vi "UHR-Fleezers Control (fpga) - 11.7.1UCBMeng5RG3.vi"() -> ()   [LabVIEW 2014]
doc: "UHR-Fleezers Instrument Control Code (fpga)"
uses:
  <vilib>/Platform/TimedLoop/XDataNode/timing_clust.ctl
  <vilib>/Platform/TimedLoop/XDataNode/nitl_modes.ctl
  <vilib>/Platform/TimedLoop/XDataNode/wakeup.ctl
  <vilib>/rvi/Emulation/niFpgaGetClockAttributes.vi
  <vilib>/rvi/Emulation/niFpgaSctlEmulationGetInTimedLoop.vi
  <vilib>/rvi/Emulation/niFpgaEmulationReportErrorSimple.vi
  <vilib>/rvi/Emulation/niFpgaProcessEmulError.vi
  <vilib>/rvi/eio/common/nirviEmuTemplateMethod_errors.vi
  <vilib>/rvi/Emulation/niFpgaCriticalErrorInLSC.vi
  <vilib>/rvi/interface/RandomDataEmulation/niFpgaRandomDataHandleErrors.vi
  <vilib>/eio/EIONode/EIONode.xnode
  <vilib>/eio/EIOMethodNode/EIOMethodNode.xnode
  <vilib>/rvi/DataTransferAndStorage/Container/XNode/niFpgaContainer.xnode
  <vilib>/rvi/interface/RandomDataEmulation/nirviRandomDataFpgaReadWriteTemplate.vi
  <vilib>/addons/control/pid/fpga.llb/XNode/niFpgaPID.xnode
  <vilib>/Platform/TimedLoop/XDataNode/XDataNode.xnode
  <vilib>/Platform/TimedLoop/XDataNode/XDNodeRunTimeDep.lvlib
panel:
  in  "Tab Control":T1(tab)=enum."Force FB"
  in  "Set 3":bool
  in  "Set 2":bool=TRUE
  in  "Set 1":bool=TRUE
  in  "Trap Pos to FIFO":bool
  in  "N of AI1 Int Acq Sets":i16=2 min=1 max=3 step=1
  out "AI Late Counter":u8
  in  "ai count":u16=400
  in  "+ phase":bool
  in  "Phase count adjustment":i16
  out "Relative phase":i16
  in  "AI to FIFO":bool
  out "BD1 Frequency Out 1":u64
  out "BD1 Frequency Out 2":u64
  out "Trap Pos FIFO Timeout":u16
  out "Trap AI FIFO Timeout":u16
  in  "Trap FIFO Set Timeout":i32
  in  "Tab Control 2":T2(tab)
  in  "FB Offset":u16
  in  "FB Multi Factor":i16
  in  "Dynamic FB (Ronen)":bool
  in  "Negate Intensity FB":bool
  in  "RD":bool
  in  "FB1 output high":i16=3000
  in  "FB1 output low":i16
  in  "D1":i16
  in  "I1":i16=5
  in  "P1":i16=10
  in  "Swap F1 and F2":bool
  in  "Cont. Scan":bool
  in  "Abort scan":bool
  in  "Cycles per step":u64
  in  "Scan BD":bool
  in  "Number of scans":u16
  in  "Scan steps":u64
  in  "Scan freq.  increment":i64
  out "Scanning":bool
  in  "Start scan":bool
  in  "OSK Bd 1":bool
  in  "Reset Bd 1":bool
  in  "PMODE":bool
  in  "Direct RF Box \nCommunication":bool
  in  "Data BD 2":u8 format="%08b"
  in  "Data BD 1":u8 format="%08b"
  in  "Address":u8 format="%02x"
  in  "Update Data":bool
  in  "FPGA Controls\n RF Box":bool
  in  "Number Interlace Cycles":u8=2 min=1 max=3
  in  "Interlace Off Parameters":u8=1 min=1 max=3
  in  "Interlace ON/OFF":bool
  out "DIO Relative phase":i16
  in  "Phase count adjustment (DIO)":i16
  in  "+ phase (DIO)":bool
  out "DIO Late Counter":u8
  in  "DIO count 1 (ticks)":u16=400
  in  "DIO count 2 (ticks)":u16=400
  in  "DIO count 3 (ticks)":u16=400
  out "AI2 Y Sum Set 2":i16
  out "AI2 Y Sum Set 1":i16
  in  "FB Setpoint Set 1":i16 min=0 step=1
  in  "FB Reset Set 1":bool
  in  "FB On/Off Set 1":bool
  in  "FB Reset Set 2":bool
  in  "FB On/Off Set 2":bool
  in  "FB Setpoint Set 2":i16 min=0 step=1
  out "Scan I":u64
  in  "Amp switch delay":u8=5
  in  "BD 2 Amplitude 1":u16
  in  "BD 1 Amplitude 1":u16
  in  "BD 2 Frequency 1":u64
  in  "BD 1 Frequency 1":u64
  in  "BD 2 Amplitude 2":u16
  in  "BD 1 Amplitude 2":u16
  in  "BD 2 Frequency 2":u64
  in  "BD 1 Frequency 2":u64
  in  "BD 2 Amplitude 3":u16
  in  "BD 1 Amplitude 3":u16
  in  "BD 2 Frequency 3":u64
  in  "BD 1 Frequency 3":u64
  in  "BD 1 Delay (ticks)":u8
  in  "BD 2 Delay (Ticks)":u8 caption="Count(Ticks)"
  in  "Next trap write delay (ticks)":u8 caption="Count(Ticks)"
  in  "FB Min frequency":u64
  in  "FB Max Frequency":u64
  in  "Dynamic Force FB (Ronen)":bool
  in  "FB2 output high":fxp<+/-,16,1>=0.999969482421875
  in  "FB2 output low":fxp<+/-,16,1>=-1.0
  in  "P2":fxp<+/-,16,8> format="%.11g"
  in  "I2":fxp<+/-,16,8>=10.0 format="%.11g"
  in  "D2":fxp<+/-,16,8> format="%.11g"
  in  "Negate Diff?":bool
  in  "Diff FB Measurement?":bool
  in  "FB Trig Integrate":u32=1
  out "TTrig?":bool
  in  "TTrig Negate Pos":bool=TRUE
  out "Trap Pos FB Int Signal":fxp<+/-,24,9> format="%.18g"
  out "Trap Pos FB Int-Norm Signal":fxp<+/-,16,1> format="%.16g"
  in  "FPGA TTrig Thresh":i64
  in  "FPGA Trap Trig":bool
  out "Trap Pos FB Action":i64
  in  "Trap Pos. FB Offset Factor":i64
  in  "Trap Pos. FB Mult Factor":i64=2
  in  "Trap Pos. FB Reset":bool
  in  "Trap Pos FB Monitor T1 or T2":bool
  in  "AI1 X Scale":u16
  in  "Trap Pos FB Int Count":u16=100
  in  "Trap Pos FB Negate Action":bool
  out "AI1 X Set 2":fxp<+/-,16,1>
  out "AI1 X Set 1":fxp<+/-,16,1>
  in  "Trap Pos. FB SP":fxp<+/-,16,1>
  in  "Force feedback":bool
  out "TTrig Sig":i64
  out "TTrig Fin Thresh":i64
  in  "B factor":fxp<+/-,32,16>
  in  "1D or 2D Scan?":bool
  in  "Abort scan (MCL)":bool
  in  "MCL Scan Axis":bool
  in  "Cont. Scan (MCL)":bool
  out "Scan I (MCL)":u64
  in  "Number of scans (MCL)":u16
  out "Scanning MCL":bool
  in  "Scan steps (MCL)":u64
  in  "Cycles per step (MCL)":u64
  in  "Scan freq.  increment (MCL)":i16
  in  "Start scan (MCL)":bool
  in  "AO2":i16
  in  "AO1":i16
  out "MCL Late Counter":u8
  in  "MCL count":u32=800
  out "MCL Relative Phase":i16
  in  "Phase count adjustment (MCL)":i16
  in  "+ phase (MCL)":bool
  out "APD2 int gate":bool
  out "APD3 out state":bool
  in  "APD Gate Operating Mode":u8 max=2 step=1
  in  "Invert APD Gate":bool
  in  "APD Gate OFF Count":u16=100
  in  "APD Gate ON Count":u16=300
  out "APD 1 Gate Late Counter":u8
  out "APD 1 Gate Relative Phase":i16
  in  "Phase count adjustment (APD 1 Gate)":i16
  in  "+ phase (APD 1 Gate)":bool
  out "APD 2 Counts 0":u32
  out "APD 2 Counts 1":u32
  out "APD 1 Counts 0":u32
  out "APD 1 Counts 1":u32
  out "APD1 out state":bool
  in  "APD AO scale factor":i16=1
  in  "APD to FIFO":bool
  in  "APD Acq Rate Count":u32=20000000
  out "APD Acq Late Counter":u8
  out "APD Acq Relative Phase":i16
  in  "Phase Count Adjustment (APD Acq)":i16
  in  "+ phase (APD Acq)":bool
  in  "Phase count adjustment (APD 2 Gate)":i16
  out "APD 2 Gate Late Counter":u8
  out "APD 2 Gate Relative Phase":i16
  in  "+ phase (APD 2 Gate)":bool
  out "APD2 out state":bool
  out "APD 3 Counts 0":u32
  out "APD 3 Counts 1":u32
  out "APD 3 Gate Late Counter":u8
  in  "Phase count adjustment (APD 3 Gate)":i16
  out "APD 3 Gate Relative Phase":i16
  in  "+ phase (APD 3 Gate)":bool
  out "APD1 int gate":bool
  out "APD3 int gate":bool
  in  "D3":i16
  in  "I3":i16=5
  in  "P3":i16=10
  in  "Green Filter Flipper":bool
  in  "Green FB Count":u16=1200
  out "Green Late Counter":u8
  out "Green FB Relative Phase":i16
  in  "Phase count adjustment (Green FB)":i16=10
  in  "+ phase (Green FB)":bool
  out "Green FB Sum":i16
  in  "Green int current ON count adj":u16=150
  in  "Current Out":u16=30000
  in  "Green FB On/Off":bool
  in  "Green FB Setpoint":i16=250 min=0 step=1
  in  "Green FB Reset":bool
  in  "Operating Mode 2":u8=2 max=2 step=1
  in  "Invert GI 2":bool
  in  "Green interlace OFF count 2":u16=900
  in  "Green interlace ON count 2":u16=300
  out "GI Late Counter 2":u8
  out "GI Relative phase 2":i16
  in  "Phase count adjustment (GI) 2":i16=20
  in  "+ phase (GI) 2":bool
  in  "Green interlace OFF count":u16=100
  out "GI Relative phase":i16
  in  "Phase count adjustment (GI)":i16
  in  "+ phase (GI)":bool
  in  "Green interlace ON count":u16=300
  out "GI Late Counter":u8
  in  "Invert GI":bool
  in  "Operating Mode":u8 max=2 step=1
  in  "+ phase (RI)":bool
  out "RI Relative phase":i16
  out "RI Late Counter":u8
  in  "Red interlace ON count":u16=300
  in  "Red interlace OFF count":u16=100
  in  "Invert RI":bool
  in  "Red Laser Operating Mode":u8 max=2 step=1
  in  "Phase count adjustment (RI)":i16
  out "Red FB Intensity":i16
  in  "RI Current Out":u16=30000
  in  "Red FB On/Off":bool
  in  "D4":i16
  in  "I4":i16=5
  in  "P4":i16=10
  in  "Red FB Setpoint":i16=250 min=0 step=1
  in  "Red FB Reset":bool
  in  "RI Operating Mode 2":u8=2 max=2 step=1
  in  "Invert RI 2":bool
  in  "Phase count adjustment (BI AO)":i16=20
  in  "Blue current ON count adj (AO)":u16=150
  in  "BI Current Out":i16=30000
  in  "Blue FB On/Off":bool
  in  "D5":i16
  in  "I5":i16=5
  in  "P5":i16=10
  in  "Blue FB Setpoint":i16=250 min=0 step=1
  in  "Blue FB Reset":bool
  in  "BI Operating Mode (AO)":u8=2 max=2 step=1
  in  "Invert BI (AO)":bool
  in  "Blue OFF count (AO)":u16=900
  in  "Blue ON count (AO)":u16=300
  out "BI Late Counter (AO)":u8
  out "BI Relative phase (AO)":i16
  in  "+ phase (BI AO)":bool
  in  "Phase count adjustment (BI D)":i16
  in  "Blue Laser Operating Mode (D)":u8 max=2 step=1
  in  "Invert BI (D)":bool
  in  "Blue interlace OFF count (D)":u16=100
  in  "Blue interlace ON count (D)":u16=300
  out "Blue Late Counter (D)":u8
  out "BI Relative phase (D)":i16
  in  "+ phase (BI D)":bool
  out "Blue Intensity":i16
  # "Only one of these can be on\nat a time:"
  # "Raster Scan AOD"
  # "1 (X)"
  # "2 (Y)"
  # "IR Intensity Feedback (RF BD 1)"
  # "FB Gains Set 1"
  # "FB output range 1"
  # "False is usual, True is external loop method"
  # "Parameters if using the external RF switching loop"
  # "Parameters if using the usual internal RF switching method"
  # "FB Triggering Excitation Laser"
  # "Trap Pos. FB Gains"
  # "Trap Pos. FB Range"
  # "AO1 (Y)"
  # "2D"
  # "1D"
  # "AO2 (X)"
  # "APD AO for aligning"
  # "Detection Loop"
  # "Green fluorescent laser digital gate interlacing loop"
  # "0 Forced ON\n1 Forced OFF\n2 Interlacing"
  # "Green FB Gains"
  # "Red fluorescent laser digital gate interlacing loop"
  # "Detection Loop"
  # "0 Forced ON\n1 Forced OFF\n2 Interlacing"
  # "Analog/FB Control Loop\n(Disabled)"
  # "Digital Control Loop"
  # "Blue laser intensity reading"
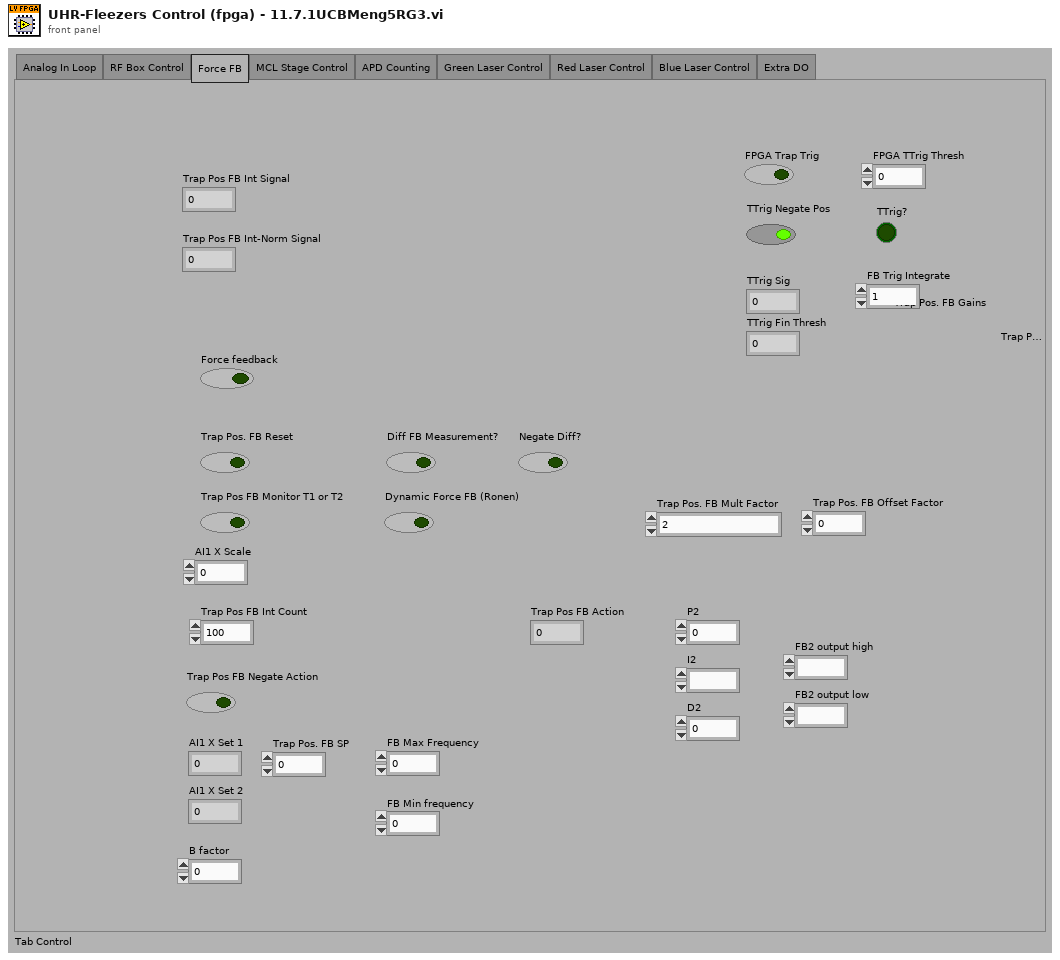
[diagram p1: front panel]
types:
  T1 = enum32{"Analog In Loop", "RF Box Control", "Force FB", "MCL Stage Control", "APD Counting", "Green Laser Control", "Red Laser Control", "Blue Laser Control", "Extra DO"}
  T2 = enum32{"Controls", "Interlacing Frequency and Amplitude Values", "Oscillate trap from memory"}
  T3 = typedef "XDNodeRunTimeDep.lvlib/timing_clust.ctl" = cluster{"Expected End [f-1]":u64, "Actual End [f-1]":u64, "Finished Late? [f-1]":bool, "Expected End [i-1]":u64, "Actual End [i-1]":u64, "Finished Late? [i-1]":bool, "Expected Start [i]":u64, "Actual Start [i]":u64, "Expected Start [f]":u64, "Actual Start [f]":u64, "Source Name":string, "Structure Name":string, "Period":i64, "Deadline":i64, "Offset":i64, "Start":i64, "Priority":i32, "Timeout":i32, "Mode":T4, "Wakeup Reason":T5, "Error":errorcluster, "Source Type":string, "Secondary Source Type":string, "Global End Time":u64, "Global Start Time":u64, "Frame Duration":u64, "Iteration Duration":u64, "Assigned CPU":i32, "I/O Scan Engine Mode":u32}
  T4 = typedef "XDNodeRunTimeDep.lvlib/nitl_modes.ctl" = enum32{"No Change", "Process missed periods, maintain original phase", "Discard missed periods, maintain original phase", "Process missed periods, ignore original phase", "Discard missed periods, ignore original phase"}
  T5 = typedef "XDNodeRunTimeDep.lvlib/wakeup.ctl" = enum32{"Normal", "Aborted", "Asynchronous wakeup", "Timing source error", "Timed loop error", "Timeout"}
  T6 = cluster{"proportional gain (Kc)":i16, "integral gain (Kc*Ts/Ti)":i16, "derivative gain (Kc*Td/Ts)":i16}
  T7 = cluster{"FB1 output high":i16, "FB1 output low":i16}
  T8 = cluster{"P2":fxp<+/-,16,8>, "I2":fxp<+/-,16,8>, "D2":fxp<+/-,16,8>}
  T9 = cluster{"FB2 output high":fxp<+/-,16,1>, "FB2 output low":fxp<+/-,16,1>}
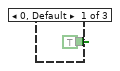
[diagram p2: hidden frame]
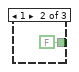
[diagram p3: hidden frame]
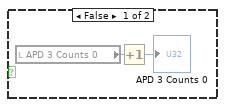
[diagram p6: hidden frame]
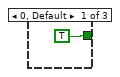
[diagram p8: hidden frame]
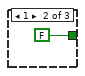
[diagram p9: hidden frame]
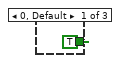
[diagram p10: hidden frame]
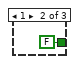
[diagram p11: hidden frame]
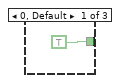
[diagram p13: hidden frame]
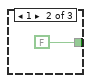
[diagram p14: hidden frame]
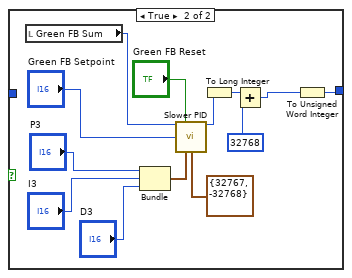
[diagram p17: hidden frame]
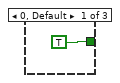
[diagram p18: hidden frame]
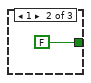
[diagram p19: hidden frame]
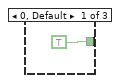
[diagram p20: hidden frame]
diagram:
  w6 = u16 0
  w7 = FALSE
  w5 = FALSE
  # "timing array current index"
  # "timing array"
  # "timing counter (phase adjusted here)"
  # "late counter"
  n1 = flat-sequence "FPGA initialization to do before running any of the loops" {
    tunnel: [u16 0 ("DIO count 3 (ticks)")] -> w4
    tunnel: [w15] -> _
    frame #0 {
      w14 = FALSE ("Enable")
      # "BD 2 (Y)"
      # "BD 1 (X)"
      # "Start up expansion chassis early\nto avoid delays later"
      # "This pin controls udclk on the RF boards.\nWhen initially configuring the boards, this pin needs to be\nconfigured as a high impedance input.  Later it will be switched\nto an output."
      # "Initial setting of DIO data and \naddress to low (before reset).  \nThis needs to happen before the other\ncontrol method loops execute."
      n2 = xnode "FPGA I/O Node"("Chassis2/Mod1/AO0"=u16 0 ("Chassis2/Mod4/AO0")) -> ("Chassis2/Mod2/AI0"=w15:i16)  [unwired: 2 in, 2 out]
      n3 = xnode "FPGA I/O Method Node"("Enable"=w14) -> ()  [unwired: 1 in, 1 out]
      n4 = xnode "FPGA I/O Method Node"("Enable"=w14) -> ()  [unwired: 1 in, 1 out]
      n5 = xnode "FPGA I/O Node"("Connector1/DIO0"=FALSE, "Connector1/DIO1"=FALSE, "Connector1/DIO2"=FALSE, "Connector1/DIO3"=FALSE, "Connector1/DIO4"=FALSE, "Connector1/DIO5"=FALSE, "Connector1/DIO6"=FALSE, "Connector1/DIO7"=FALSE, "Connector1/DIO8"=FALSE, "Connector1/DIO9"=FALSE, "Connector1/DIO10"=FALSE, "Connector1/DIO11"=FALSE, "Connector1/DIO12"=FALSE, "Connector1/DIO13"=FALSE, "Connector1/DIO15"=FALSE, "Connector1/DIO20"=FALSE, "Connector1/DIO21"=FALSE, "Connector1/DIO22"=FALSE, "Connector1/DIO23"=FALSE, "Connector1/DIO24"=FALSE, "Connector1/DIO25"=FALSE, "Connector1/DIO26"=FALSE, "Connector1/DIO27"=FALSE, "Connector1/DIO14"=FALSE) -> ()  [unwired: 24 in, 24 out]
    }
  }
  n6 = local read "AO1"() -> (w12:i16)
  n7 = local read "AO2"() -> (w11:i16)
  n8 = node-c288() -> (w10:T3)  [unwired: 1 in]
  n9 = disable-structure shown="Disabled" {
    disable-tunnel: w4 -> [w42 _]
    frame Disabled {
      n10 = while "Excitation laser intensity feedback measurement (all lasers)" {
        shift-right: [w43] -> _
        shift-left: w42 -> [w48]
        stop <- FALSE stop-if-true
        n11 = flat-sequence {
          tunnel: w48 -> [w50]
          tunnel: [w51] -> w46
          tunnel: [w50] -> w44
          tunnel: [w57] -> w47
          tunnel: w46 -> [w57]
          tunnel: [w56] -> w45
          tunnel: w44 -> [w56]
          tunnel: [w69] -> w43
          tunnel: w47 -> [w80]
          tunnel: w45 -> [w77]
          frame #0 {
            n12 = call "Loop Timer9"("Count(Ticks)"=w50) -> ("Tick Count(Ticks)"=w51:u16)
          }
          frame #1 {
            # "Design note:\n\nAll lasers need to be measured at the same \ntime because the AI expansion module\ncannot independently time the measurements\nwithin our requirements: their is dead time.\n\nThis probably wouldn't be an issue with the built\nin AI on the fpga board itself."
            n13 = xnode "FPGA I/O Node"("Connector1/DIO35"=TRUE) -> ("Chassis2/Mod2/AI2"=→"Blue Intensity":i16, "Chassis2/Mod2/AI1"=→"Red FB Intensity":i16, "Chassis2/Mod2/AI0"=→"Green FB Sum":i16)  [unwired: 4 in, 4 out]
          }
          frame #2 {
            n14 = feedback-in #1(w80) -> ()
            n15 = feedback #1(w80) -> (w79:u16)
            n16 = Subtract(x=w80, y=w79) -> (x-y=w78:u16)
            n17 = xnode "FPGA I/O Node"("Connector1/DIO35"=FALSE) -> ()  [unwired: 1 in, 1 out]
            n18 = Subtract(x=w78, y=w77) -> (x-y=w59:u16)
            n19 = Subtract(x="Green FB Count", y=w59) -> (x-y=w73:u16)
            n20 = Number To Boolean Array(number=w59) -> (Boolean array=w60:bool[])
            n21 = Or Array Elements(Boolean array=w60) -> (logical OR=w58:bool)
            n22 = Boolean To (0,1)(Boolean="+ phase (Green FB)") -> (0, 1=w71:i16)
            n23 = Boolean To (0,1)(Boolean=w58) -> (0, 1=w65:i16)
            n24 = Multiply(x=w71, y="Phase count adjustment (Green FB)") -> (x*y=w66:i16)
            n25 = Add(x=w73, y=w66) -> (x+y=w69:u16)
            n26 = To Unsigned Byte Integer(number=w65) -> (unsigned 8bit integer=w62:u8)
            n27 = feedback #2(i16 0) -> (w68:i16)
            n28 = Subtract(x=w68, y=w66) -> (x-y=w67:i16)
            "Green FB Relative Phase" <- w67
            n29 = feedback-in #2(w67) -> ()
            n30 = feedback #3(u8 0) -> (w63:u8)
            n31 = Add(x=w62, y=w63) -> (x+y=w61:u8)
            "Green Late Counter" <- w61
            n32 = feedback-in #3(w61) -> ()
          }
        }
      }
    }
    frame Enabled {
    }
  }
  n33 = To Unsigned Long Integer(number=w4) -> (unsigned 32bit integer=w8:u32)
  n34 = timed-loop "RF box board DIO control: control bits" {
    timing: w10 -> [_]
    timing-out: [_] -> w9
    tunnel: [w83] -> _
    tunnel: w4 -> [w83]
    stop <- FALSE stop-if-true
    n35 = xnode "FPGA I/O Node"("Connector1/DIO16"="RD", "Connector1/DIO17"="PMODE", "Connector1/DIO18"="OSK Bd 1", "Connector1/DIO19"="Reset Bd 1", "Connector0/DIO3"="Green Filter Flipper") -> ()  [unwired: 5 in, 5 out]
  }
  n36 = while "RF box board direct communication loop" {
    tunnel: w4 -> [_]
    stop <- FALSE stop-if-true
    n37 = case "Whether to use direct communication method (only use one method at a time)" shown="True" "Direct RF Box \nCommunication" {
      frame False {
      }
      frame True {
        n38 = case shown="True" "Update Data" {
          frame False {
          }
          frame True {
            n39 = flat-sequence {
              frame #0 {
                n40 = First Call?() -> (First Call?: T/F=w93:bool)
                n41 = case shown="True" w93 {
                  frame False {
                  }
                  frame True {
                    # "If first time data updated, be sure to set WR high\nbefore setting data and address bits."
                    n42 = flat-sequence {
                      frame #0 {
                        n43 = xnode "FPGA I/O Node"("Connector1/DIO15"=TRUE) -> ()  [unwired: 1 in, 1 out]
                      }
                      frame #1 {
                        n44 = call "Wait"("Count(Ticks)"=u8 40 ("DO Delay 3 (Ticks)")) -> ()  [unwired: 1 out]
                      }
                    }
                  }
                }
              }
              frame #1 {
                n45 = Number To Boolean Array(number="Address") -> (Boolean array=w142:bool[])
                n46 = Number To Boolean Array(number="Data BD 1") -> (Boolean array=w143:bool[])
                n47 = Number To Boolean Array(number="Data BD 2") -> (Boolean array=w112:bool[])
                n48 = Index Array(array=w143, index=7) -> (element=w127:bool)
                n49 = Index Array(array=w143, index=6) -> (element=w126:bool)
                n50 = Index Array(array=w143, index=5) -> (element=w125:bool)
                n51 = Index Array(array=w143, index=4) -> (element=w124:bool)
                n52 = Index Array(array=w143, index=3) -> (element=w123:bool)
                n53 = Index Array(array=w143, index=2) -> (element=w122:bool)
                n54 = Index Array(array=w143, index=1) -> (element=w121:bool)
                n55 = Index Array(array=w143, index=0) -> (element=w120:bool)
                n56 = Index Array(array=w142, index=5) -> (element=w119:bool)
                n57 = Index Array(array=w142, index=4) -> (element=w118:bool)
                n58 = Index Array(array=w142, index=3) -> (element=w117:bool)
                n59 = Index Array(array=w142, index=2) -> (element=w116:bool)
                n60 = Index Array(array=w142, index=1) -> (element=w115:bool)
                n61 = Index Array(array=w142, index=0) -> (element=w114:bool)
                n62 = Index Array(array=w112, index=7) -> (element=w103:bool)
                n63 = Index Array(array=w112, index=6) -> (element=w102:bool)
                n64 = Index Array(array=w112, index=5) -> (element=w101:bool)
                n65 = Index Array(array=w112, index=4) -> (element=w100:bool)
                n66 = Index Array(array=w112, index=3) -> (element=w99:bool)
                n67 = Index Array(array=w112, index=2) -> (element=w98:bool)
                n68 = Index Array(array=w112, index=1) -> (element=w97:bool)
                n69 = Index Array(array=w112, index=0) -> (element=w96:bool)
                n70 = xnode "FPGA I/O Node"("Connector1/DIO0"=w127, "Connector1/DIO1"=w126, "Connector1/DIO2"=w125, "Connector1/DIO3"=w124, "Connector1/DIO4"=w123, "Connector1/DIO5"=w122, "Connector1/DIO6"=w121, "Connector1/DIO7"=w120, "Connector1/DIO8"=w119, "Connector1/DIO9"=w118, "Connector1/DIO10"=w117, "Connector1/DIO11"=w116, "Connector1/DIO12"=w115, "Connector1/DIO13"=w114, "Connector1/DIO20"=w103, "Connector1/DIO21"=w102, "Connector1/DIO22"=w101, "Connector1/DIO23"=w100, "Connector1/DIO24"=w99, "Connector1/DIO25"=w98, "Connector1/DIO26"=w97, "Connector1/DIO27"=w96) -> ()  [unwired: 22 in, 22 out]
              }
              frame #2 {
                # "wait and then apply write signal"
                n71 = call "Wait2"("Count(Ticks)"=u8 40 ("DO Delay 1 (Ticks)")) -> ()  [unwired: 1 out]
              }
              frame #3 {
                # "sending bit low writes data to board buffer"
                n72 = xnode "FPGA I/O Node"("Connector1/DIO15"=FALSE) -> ()  [unwired: 1 in, 1 out]
              }
              frame #4 {
                # "wait then return write signal"
                n73 = call "Wait3"("Count(Ticks)"=u8 40 ("DO Delay 2 (Ticks)")) -> ()  [unwired: 1 out]
              }
              frame #5 {
                # "sending bit high makes ready to\nwrite more data"
                n74 = xnode "FPGA I/O Node"("Connector1/DIO15"=TRUE) -> ()  [unwired: 1 in, 1 out]
              }
            }
          }
        }
      }
    }
  }
  n75 = while "RF box board DIO control: parallel communication" {
    shift-right: [w162] -> _
    shift-left: w4 -> [w161]
    shift-right: [w160] -> _
    shift-left: FALSE ("Swap F1 and F2") -> [w159]
    shift-right: [w154] -> _
    shift-left: u16 0 -> [w155]
    shift-right: [w152] -> _
    shift-left: u16 0 -> [w153]
    shift-right: [w150] -> _
    shift-left: u64 0 -> [w151]
    stop <- FALSE stop-if-true
    n76 = flat-sequence {
      tunnel: w159 -> [w166]
      tunnel: w161 -> [w164]
      tunnel: [w166] -> w158
      tunnel: [w165] -> w157
      tunnel: [w164] -> w156
      tunnel: [w178] -> w162
      tunnel: [w177] -> w160
      tunnel: w158 -> [w176]
      tunnel: w157 -> [w174]
      tunnel: w156 -> [w173]
      tunnel: w155 -> [w172]
      tunnel: [w171] -> w154
      tunnel: w153 -> [w170]
      tunnel: [w169] -> w152
      tunnel: w151 -> [w168]
      tunnel: [w167] -> w150
      frame #0 {
        n77 = call "Loop Timer"("Count(Ticks)"=w164) -> ("Tick Count(Ticks)"=w165:u16)
      }
      frame #1 {
        n78 = flat-sequence {
          tunnel: ["FPGA Controls\n RF Box"] -> w175
          tunnel: w176 -> [w179]
          tunnel: [w244] -> w178
          tunnel: [w257] -> w177
          tunnel: w175 -> [w256]
          tunnel: w174 -> [w250]
          tunnel: w173 -> [w247]
          tunnel: w172 -> [w213]
          tunnel: [w212] -> w171
          tunnel: w170 -> [w209]
          tunnel: [w208] -> w169
          tunnel: w168 -> [w207]
          tunnel: [w206] -> w167
          frame #0 {
            n79 = case shown="True" "FPGA Controls\n RF Box" {
              tunnel: w179 -> [_ w181]
              frame False {
              }
              frame True {
                n80 = flat-sequence {
                  tunnel: w181 -> [w191]
                  frame #0 {
                    n81 = First Call?() -> (First Call?: T/F=w182:bool)
                    n82 = case shown="True" w182 {
                      frame False {
                      }
                      frame True {
                        # "BD 2"
                        # "BD 1"
                        # "If first time data updated, be sure to set WR high and UDCLK low\nbefore setting data and address bits."
                        n83 = xnode "FPGA I/O Method Node"("Enable"=TRUE) -> ("FPGA I/O Out"=w184:refnum<k21>)  [unwired: 1 in]
                        n84 = xnode "FPGA I/O Method Node"("Enable"=TRUE) -> ("FPGA I/O Out"=w187:refnum<k21>)  [unwired: 1 in]
                        n85 = xnode "FPGA I/O Node"("Connector1/DIO15"=TRUE) -> ()  [unwired: 1 in, 1 out]
                        n86 = xnode "FPGA I/O Node"("I/O Item"=FALSE ("Connector1/DIO30"), "FPGA I/O In"=w184) -> ()  [unwired: 1 out]
                        n87 = xnode "FPGA I/O Node"("I/O Item"=FALSE ("Connector1/DIO30"), "FPGA I/O In"=w187) -> ()  [unwired: 1 out]
                      }
                    }
                  }
                  frame #1 {
                    n88 = case shown="False" FALSE {
                      tunnel: w191 -> [w193 _]
                      frame False {
                        # "Usual operation"
                        n89 = disable-structure shown="Disabled" {
                          disable-tunnel: w193 -> [w195 _]
                          disable-tunnel: "Amp switch delay" -> [w194 _]
                          frame Disabled {
                            n90 = flat-sequence "BD 2 (Y)" {
                              tunnel: w195 -> [w197]
                              tunnel: w194 -> [w198]
                              frame #0 {
                                n91 = call "Wait7"("Count(Ticks)"="BD 2 Delay (Ticks)") -> ()  [unwired: 1 out]
                              }
                              frame #1 {
                                # "switch frequency"
                                n92 = xnode "FPGA I/O Node"("Connector1/DIO37"=w197) -> ()  [unwired: 1 in, 1 out]
                              }
                              frame #2 {
                                # "~5 ticks is usual"
                                n93 = call "Wait5"("Count(Ticks)"=w198) -> ()  [unwired: 1 out]
                              }
                              frame #3 {
                                # "this switches amplitude"
                                # "switch amplitude"
                                # "send udclk high"
                                n94 = xnode "FPGA I/O Node"("Connector1/DIO29"=TRUE ("Connector1/DIO15")) -> ()  [unwired: 1 in, 1 out]
                              }
                              frame #4 {
                                # "reset to be ready for next\ncycle"
                                # "send udclk low"
                                n95 = xnode "FPGA I/O Node"("Connector1/DIO29"=FALSE ("Connector1/DIO15")) -> ()  [unwired: 1 in, 1 out]
                              }
                            }
                          }
                          frame Enabled {
                          }
                        }
                        n96 = flat-sequence "BD 1 (X)" {
                          tunnel: w193 -> [w202]
                          tunnel: "Amp switch delay" -> [w203]
                          frame #0 {
                            n97 = call "Wait6"("Count(Ticks)"="BD 1 Delay (ticks)") -> ()  [unwired: 1 out]
                          }
                          frame #1 {
                            # "switch frequency"
                            n98 = xnode "FPGA I/O Node"("Connector1/DIO36"=w202) -> ()  [unwired: 1 in, 1 out]
                          }
                          frame #2 {
                            # "~5 ticks is usual"
                            n99 = call "Wait4"("Count(Ticks)"=w203) -> ()  [unwired: 1 out]
                          }
                          frame #3 {
                            # "this switches amplitude"
                            # "switch amplitude"
                            # "send udclk high"
                            n100 = xnode "FPGA I/O Node"("Connector1/DIO30"=TRUE ("Connector1/DIO15")) -> ()  [unwired: 1 in, 1 out]
                          }
                          frame #4 {
                            # "reset to be ready for next\ncycle"
                            # "send udclk low"
                            n101 = xnode "FPGA I/O Node"("Connector1/DIO30"=FALSE ("Connector1/DIO15")) -> ()  [unwired: 1 in, 1 out]
                          }
                        }
                      }
                      frame True {
                        # "Operation when you need a long delay for either X or Y to synchonize AOD light out phase (> ~100 ticks)."
                        # "Trigger the external loop by sending the boolean FSK value through a FIFO"
                      }
                    }
                  }
                }
              }
            }
          }
          frame #1 {
            # "This is the prior cycle's on time"
            # "increment timing\nindex, reset to 0 if \nend of matrix"
            # "Reset to begginning (1) when number of cycles reached."
            # "timing index"
            # "build byte stacks for writing data\n(must correspond to addresses array constant)"
            # "Timing housekeeping"
            # "Adjust phase if late\n(maintains constant phase relationship between cycles)"
            n102 = Bundle("FB1 output high"="FB1 output high", "FB1 output low"="FB1 output low") -> (w217:T7)  [unwired: 1 in]
            n103 = Bundle("P1"="P1", "I1"="I1", "D1"="D1") -> (w218:cluster{"P1":i16, "I1":i16, "D1":i16})  [unwired: 1 in]
            n104 = feedback #4(u8 0 ("t")) -> (w253:u8)
            n105 = Increment(x=w253) -> (x+1=w296:u8)
            n106 = Increment(x="Number Interlace Cycles") -> (x+1=w291:u8)
            n107 = Equal?(x=w296, y=w291) -> (x = y?=w298:bool)
            n108 = Select(t=u8 1, s=w298, f=w296) -> (s? t:f=w252:u8)
            n109 = feedback-in #4(w252) -> ()
            n110 = Increment(x=w252) -> (x+1=w293:u8)
            n111 = Equal?(x=w293, y=w291) -> (x = y?=w294:bool)
            n112 = Select(t=u8 1, s=w294, f=w293) -> (s? t:f=w290:u8)
            n113 = Select(t=w290, s="Interlace ON/OFF", f="Interlace Off Parameters") -> (s? t:f=w216:u8)
            n114 = case shown="1, Default" w216 {
              tunnel: [w340 w595 "BD 1 Frequency 3"] -> w286
              tunnel: [w390 "BD 2 Frequency 2" "BD 2 Frequency 3"] -> w275
              tunnel: ["BD 2 Amplitude 1" "BD 2 Amplitude 2" "BD 2 Amplitude 3"] -> w232
              tunnel: [w352 w589 "BD 1 Amplitude 3"] -> w235
              tunnel: w218 -> [w359 w597 _]
              tunnel: w217 -> [w360 w596 _]
              tunnel: "Negate Intensity FB" -> [w358 w593 _]
              tunnel: "Dynamic FB (Ronen)" -> [w357 w592 _]
              tunnel: w213 -> [w353 w591 w643]
              tunnel: [w352 w591 w643] -> w212
              tunnel: "FB Multi Factor" -> [w351 w588 _]
              tunnel: "FB Offset" -> [w350 w587 _]
              tunnel: w209 -> [w349 w590 w642]
              tunnel: [w349 w589 w642] -> w208
              tunnel: w207 -> [w348 w586 w641]
              tunnel: [w340 w586 w641] -> w206
              frame 1, Default {
                w374 = fxp<+/-,24,9> 0.0 ("AI1 X Set 2")
                w368 = u16 0
                w386 = u64 0 ("f")
                # "Added by Ronen -\nUpper and Lower \nLimits for the FB \ngenerated frequency\nto avoid losing bead \nwhen tether breaks"
                # "Changed by Ronen - correction \nby PID is now implemented not on \nthe Base BD1 frequency but on the last\nfrequency sent."
                # "BD1 Amp 1"
                # "Changed by Ronen-\n FB changed \nso that value from PID is added to\nlast amplitude sent to board. Correction\nValue can be scaled down same as the force\nFB value."
                # "This signal integration happens no matter what\nso that correct setpoints can be chosen before \nturning on the FB."
                # "Trap 1"
                n115 = local read "AI1 X Set 2"() -> (w343:fxp<+/-,16,1>)
                n116 = local read "AI1 X Set 1"() -> (w371:fxp<+/-,16,1>)
                n117 = local read "Scanning"() -> (w391:bool)
                n118 = Multiply(x=w343, y="B factor") -> (x*y=w341:fxp<+/-,48,17>)
                n119 = Or(x=w391, y="Start scan") -> (x .or. y?=w384:bool)
                n120 = case shown="True" "Diff FB Measurement?" {
                  tunnel: w341 -> [w409 w418]
                  tunnel: w371 -> [w408 w419]
                  tunnel: [w406 w410] -> w372
                  frame False {
                    n121 = Select(t=w408, s="Trap Pos FB Monitor T1 or T2", f=w409) -> (s? t:f=w406:fxp<+/-,48,17>)
                  }
                  frame True {
                    n122 = Subtract(x=w419, y=w418) -> (x-y=w411:fxp<+/-,48,17>)
                    n123 = Not(x="Negate Diff?") -> (.not. x?=w417:bool)
                    n124 = Boolean To (0,1)(Boolean="Negate Diff?") -> (0, 1=w415:i16)
                    n125 = Boolean To (0,1)(Boolean=w417) -> (0, 1=w416:i16)
                    n126 = Negate(x=w415) -> (-x=w414:i16)
                    n127 = Add(x=w414, y=w416) -> (x+y=w412:i16)
                    n128 = Multiply(x=w412, y=w411) -> (x*y=w410:fxp<+/-,63,32>)
                  }
                }
                n129 = Not(x="Abort scan") -> (.not. x?=w382:bool)
                n130 = And(x=w382, y=w384) -> (x .and. y?=w381:bool)
                n131 = case "For raster scanning" shown="True" w381 {
                  tunnel: [u64 0 w545] -> w387
                  tunnel: "Start scan" -> [_ w530]
                  frame False {
                    n132 = local write "Scanning"(FALSE ("scanning")) -> ()
                  }
                  frame True {
                    w514 = i64 0
                    w513 = u64 0
                    # "scan incr."
                    # "freq. incr. mult."
                    # "count steps"
                    # "count number of cycles"
                    n133 = feedback #5(w513) -> (w542:u64)
                    n134 = Select(t=w513, s=w530, f=w542) -> (s? t:f=w544:u64)
                    n135 = Increment(x=w544) -> (x+1=w541:u64)
                    n136 = Greater?(x="Cycles per step", y=w541) -> (0:w523:bool)
                    n137 = Select(t=w541, s=w523, f=w513) -> (s? t:f=w540:u64)
                    n138 = feedback-in #5(w540) -> ()
                    n139 = feedback #6(w513) -> (w539:u64)
                    n140 = Select(t=w513, s=w530, f=w539) -> (s? t:f=w534:u64)
                    n141 = Increment(x=w534) -> (x+1=w538:u64)
                    n142 = Add(x="Scan steps", y="Scan steps") -> (x+y=w537:u64)
                    n143 = Select(t=w534, s=w523, f=w538) -> (s? t:f=w518:u64)
                    n144 = Greater?(x=w537, y=w518) -> (0:w517:bool)
                    n145 = Select(t=w518, s=w517, f=w513) -> (s? t:f=w535:u64)
                    n146 = feedback-in #6(w535) -> ()
                    n147 = Equal?(x="Scan steps", y=w518) -> (x = y?=w522:bool)
                    n148 = Greater?(x="Scan steps", y=w534) -> (0:w533:bool)
                    n149 = feedback #7(w514) -> (w536:i64)
                    n150 = Select(t=w514, s=w530, f=w536) -> (s? t:f=w520:i64)
                    n151 = Increment(x=w520) -> (x+1=w532:i64)
                    n152 = Decrement(x=w520) -> (x-1=w531:i64)
                    n153 = Select(t=w532, s=w533, f=w531) -> (s? t:f=w521:i64)
                    n154 = Select(t=w520, s=w522, f=w521) -> (s? t:f=w519:i64)
                    n155 = Select(t=w520, s=w523, f=w519) -> (s? t:f=w515:i64)
                    n156 = Select(t=w515, s=w517, f=w514) -> (s? t:f=w516:i64)
                    n157 = feedback-in #7(w516) -> ()
                    n158 = feedback #8(w513) -> (w529:u64)
                    n159 = Select(t=w513, s=w530, f=w529) -> (s? t:f=w525:u64)
                    n160 = Increment(x=w525) -> (x+1=w526:u64)
                    n161 = Select(t=w525, s=w517, f=w526) -> (s? t:f=w524:u64)
                    n162 = Greater?(x="Number of scans", y=w524) -> (0:w510:bool)
                    n163 = Multiply(x="Scan freq.  increment", y=w520) -> (x*y=w545:i64)
                    n164 = Select(t=TRUE, s="Cont. Scan", f=w510) -> (s? t:f=w509:bool)
                    "Scanning" <- w509
                    n165 = Select(t=w524, s=w509, f=w513) -> (s? t:f=w527:u64)
                    n166 = feedback-in #8(w527) -> ()
                    n167 = Increment(x=w524) -> (x+1=→"Scan I":u64)
                  }
                }
                n168 = feedback #9(w368) -> (w367:u16)
                n169 = Increment(x=w367) -> (x+1=w369:u16)
                n170 = Greater Or Equal?(x=w369, y="Trap Pos FB Int Count") -> (x >= y?=w347:bool)
                n171 = Select(t=w368, s=w347, f=w369) -> (s? t:f=w370:u16)
                n172 = feedback-in #9(w370) -> ()
                n173 = feedback #10(w374) -> (w373:fxp<+/-,24,9>)
                n174 = Add(x=w372, y=w373) -> (x+y=w366:fxp<+/-,24,9>)
                n175 = case "For intensity feedback" shown="True" "FB On/Off Set 1" {
                  tunnel: w353 -> [_ w550]
                  tunnel: ["BD 1 Amplitude 1" w556] -> w352
                  tunnel: w360 -> [_ w557]
                  tunnel: w359 -> [_ w558]
                  tunnel: w358 -> [_ w555]
                  tunnel: w357 -> [_ w554]
                  tunnel: w351 -> [_ w549]
                  tunnel: w350 -> [_ w548]
                  frame False {
                  }
                  frame True {
                    n176 = local read "AI2 Y Sum Set 1"() -> (w552:i16)
                    n177 = case shown="True" w554 {
                      tunnel: w558 -> [w564 w578]
                      tunnel: w557 -> [w565 w577]
                      tunnel: [w559 w576] -> w556
                      tunnel: w555 -> [_ w575]
                      tunnel: "FB Setpoint Set 1" -> [w563 w574]
                      tunnel: w552 -> [w562 w573]
                      tunnel: "FB Reset Set 1" -> [w561 w572]
                      tunnel: w550 -> [_ w571]
                      tunnel: w549 -> [_ w569]
                      tunnel: w548 -> [_ w567]
                      frame False {
                        n178 = call "Slower PID.vi"("process variable"=w562, "reset?"=w561, "setpoint"=w563, "PID gains (x 2^8)"=w564, "output range"=w565) -> ("output"=w560:i16)  [unwired: 10 out]
                        n179 = To Unsigned Word Integer(number=w560) -> (unsigned 16bit integer=w559:u16)
                      }
                      frame True {
                        n180 = call "Slower PID.vi"("process variable"=w573, "reset?"=w572, "setpoint"=w574, "PID gains (x 2^8)"=w578, "output range"=w577) -> ("output"=w579:i16)  [unwired: 10 out]
                        n181 = To Unsigned Word Integer(number=w579) -> (unsigned 16bit integer=w570:u16)
                        n182 = Scale By Power Of 2(n=w569, x=w570) -> (x*2^n=w568:u16)
                        n183 = Add(x=w568, y=w567) -> (x+y=w566:u16)
                        n184 = case shown="True" w575 {
                          tunnel: w566 -> [w582 w584]
                          tunnel: w571 -> [w580 w585]
                          tunnel: [w581 w583] -> w576
                          frame False {
                            n185 = Add(x=w580, y=w582) -> (x+y=w581:u16)
                          }
                          frame True {
                            n186 = Subtract(x=w585, y=w584) -> (x-y=w583:u16)
                          }
                        }
                      }
                    }
                  }
                }
                n187 = Select(t=w374, s=w347, f=w366) -> (s? t:f=w377:fxp<+/-,24,9>)
                n188 = feedback-in #10(w377) -> ()
                n189 = Divide(x=w366, y="Trap Pos FB Int Count") -> (x/y=w361:fxp<+/-,16,1>)
                n190 = feedback #11(fxp<+/-,24,9> 0.0 ("AI1 X Set 2")) -> (w378:fxp<+/-,24,9>)
                n191 = Select(t=w366, s=w347, f=w378) -> (s? t:f=w379:fxp<+/-,24,9>)
                "Trap Pos FB Int Signal" <- w379
                n192 = feedback-in #11(w379) -> ()
                n193 = feedback #12(fxp<+/-,16,1> 0.0 ("Trap Pos FB Int-Norm Signal")) -> (w363:fxp<+/-,16,1>)
                n194 = Select(t=w361, s=w347, f=w363) -> (s? t:f=w362:fxp<+/-,16,1>)
                "Trap Pos FB Int-Norm Signal" <- w362
                n195 = feedback-in #12(w362) -> ()
                n196 = case "For position feedback" shown="True" "Force feedback" {
                  tunnel: [i64 0 w425] -> w356
                  tunnel: w361 -> [_ w422]
                  tunnel: w347 -> [_ w421]
                  frame False {
                  }
                  frame True {
                    n197 = feedback #13(i64 0) -> (w424:i64)
                    n198 = case shown="True" w421 {
                      tunnel: [w426 w440] -> w425
                      tunnel: w424 -> [w426 _]
                      tunnel: w422 -> [_ w434]
                      frame False {
                      }
                      frame True {
                        w444 = u32 0
                        n199 = Bundle("P2"="P2", "I2"="I2", "D2"="D2") -> (w430:T8)  [unwired: 1 in]
                        n200 = Bundle("FB2 output high"="FB2 output high", "FB2 output low"="FB2 output low") -> (w427:T9)  [unwired: 1 in]
                        n201 = xnode ("PID")("process variable"=w434, "reset?"="Trap Pos. FB Reset", "setpoint"="Trap Pos. FB SP", "PID gains"=w430, "output range"=w427) -> ("output"=w456:fxp<+/-,16,1>)
                        n202 = Negate(x=w456) -> (-x=w455:fxp<+/-,17,2>)
                        n203 = Select(t=w455, s="Trap Pos FB Negate Action", f=w456) -> (s? t:f=w452:fxp<+/-,17,2>)
                        n204 = Scale By Power Of 2(n=u32 15, x=u32 1) -> (x*2^n=w449:u32)
                        n205 = Multiply(x=w452, y=w449) -> (x*y=w448:fxp<+/-,17,17>)
                        n206 = To Quad Integer(1:w448) -> (0:w460:i64)
                        "Trap Pos FB Action" <- w460
                        n207 = Multiply(x=w460, y="Trap Pos. FB Mult Factor") -> (x*y=w458:i64)
                        n208 = Add(x=w458, y="Trap Pos. FB Offset Factor") -> (x+y=w440:i64)
                        n209 = feedback #14() -> (w441:i64)  [unwired: 1 in]
                        n210 = Add(x=w440, y=w441) -> (x+y=w438:i64)
                        n211 = feedback #15(w444) -> (w446:u32)
                        n212 = Increment(x=w446) -> (x+1=w435:u32)
                        n213 = Greater Or Equal?(x=w435, y="FB Trig Integrate") -> (x >= y?=w436:bool)
                        n214 = Select(t=i64 0, s=w436, f=w438) -> (s? t:f=w442:i64)
                        n215 = feedback-in #14(w442) -> ()
                        n216 = Select(t=w444, s=w436, f=w435) -> (s? t:f=w445:u32)
                        n217 = feedback-in #15(w445) -> ()
                        n218 = And(x=w436, y="FPGA Trap Trig") -> (x .and. y?=w443:bool)
                        n219 = case "Trap FB trigger excitation laser ON" shown="True" w443 {
                          tunnel: w438 -> [_ w464]
                          tunnel: w435 -> [_ w462]
                          frame False {
                          }
                          frame True {
                            n220 = Not(x="TTrig Negate Pos") -> (.not. x?=w471:bool)
                            n221 = Boolean To (0,1)(Boolean="TTrig Negate Pos") -> (0, 1=w469:i16)
                            n222 = Boolean To (0,1)(Boolean=w471) -> (0, 1=w470:i16)
                            n223 = Negate(x=w469) -> (-x=w468:i16)
                            n224 = Add(x=w468, y=w470) -> (x+y=w467:i16)
                            n225 = Multiply(x=w467, y=w464) -> (x*y=w466:i64)
                            "TTrig Sig" <- w466
                            n226 = Multiply(x="FPGA TTrig Thresh", y=w462) -> (x*y=w463:i64)
                            "TTrig Fin Thresh" <- w463
                            n227 = Greater Or Equal?(x=w466, y=w463) -> (x >= y?=w465:bool)
                            n228 = case shown="True" w465 {
                              frame False {
                              }
                              frame True {
                                w474 = TRUE ("Green FB On/Off")
                                w476 = u8 2 ("Operating Mode")
                                n229 = local write "Operating Mode 2"(w476) -> ()
                                n230 = local write "Operating Mode"(w476) -> ()
                                n231 = local write "Green FB On/Off"(w474) -> ()
                                n232 = local write "FPGA Trap Trig"(FALSE ("FPGA Trap Trig")) -> ()
                                "TTrig?" <- w474
                              }
                            }
                          }
                        }
                      }
                    }
                    n233 = feedback-in #13(w425) -> ()
                  }
                }
                n234 = And(x="Force feedback", y="Dynamic Force FB (Ronen)") -> (x .and. y?=w337:bool)
                n235 = case shown="True" w337 {
                  tunnel: w356 -> [w397 w401]
                  tunnel: [w396 w400] -> w354
                  tunnel: w348 -> [_ w399]
                  tunnel: w347 -> [_ w398]
                  frame False {
                    # "(BD1 Frequency 1)"
                    n236 = Add(x="BD 1 Frequency 1", y=w397) -> (x+y=w396:u64)
                  }
                  frame True {
                    n237 = case shown="True" w398 {
                      tunnel: w401 -> [_ w405]
                      tunnel: [w402 w404] -> w400
                      tunnel: w399 -> [w402 w403]
                      frame False {
                      }
                      frame True {
                        n238 = Add(x=w403, y=w405) -> (x+y=w404:u64)
                      }
                    }
                  }
                }
                n239 = Select(t=w386, s="Scan BD", f=w387) -> (s? t:f=w385:u64)
                n240 = Select(t=w387, s="Scan BD", f=w386) -> (s? t:f=w388:u64)
                n241 = Add(x=w385, y="BD 2 Frequency 1") -> (x+y=w390:u64)
                n242 = Compound Arithmetic op=ADD(i64 0 ("f"), w354, w388) -> (w346:u64)
                n243 = In Range and Coerce(upper limit="FB Max Frequency", x=w346, lower limit="FB Min frequency") -> (coerced(x)=w340:u64)  [unwired: 1 out]
                "BD1 Frequency Out 1" <- w340
              }
              frame 2 {
                # "Trap 2"
                n244 = case shown="True" "FB On/Off Set 2" {
                  tunnel: ["BD 1 Amplitude 2" w607] -> w589
                  tunnel: w590 -> [_ w605]
                  tunnel: w597 -> [_ w610]
                  tunnel: w596 -> [_ w609]
                  tunnel: w593 -> [_ w608]
                  tunnel: w592 -> [_ w606]
                  tunnel: w588 -> [_ w604]
                  tunnel: w587 -> [_ w603]
                  frame False {
                  }
                  frame True {
                    n245 = local read "AI2 Y Sum Set 2"() -> (w612:i16)
                    n246 = case shown="False" w606 {
                      tunnel: "FB Setpoint Set 2" -> [w618 w634]
                      tunnel: w612 -> [w619 w633]
                      tunnel: "FB Reset Set 2" -> [w620 w632]
                      tunnel: w610 -> [w616 w630]
                      tunnel: w609 -> [w617 w629]
                      tunnel: w608 -> [_ w628]
                      tunnel: [w614 w627] -> w607
                      tunnel: w605 -> [_ w626]
                      tunnel: w604 -> [_ w625]
                      tunnel: w603 -> [_ w622]
                      frame False {
                        n247 = call "Slower PID.vi"("process variable"=w619, "reset?"=w620, "setpoint"=w618, "PID gains (x 2^8)"=w616, "output range"=w617) -> ("output"=w615:i16)  [unwired: 10 out]
                        n248 = To Unsigned Word Integer(number=w615) -> (unsigned 16bit integer=w614:u16)
                      }
                      frame True {
                        n249 = call "Slower PID.vi"("process variable"=w633, "reset?"=w632, "setpoint"=w634, "PID gains (x 2^8)"=w630, "output range"=w629) -> ("output"=w631:i16)  [unwired: 10 out]
                        n250 = To Unsigned Word Integer(number=w631) -> (unsigned 16bit integer=w624:u16)
                        n251 = Scale By Power Of 2(n=w625, x=w624) -> (x*2^n=w623:u16)
                        n252 = Add(x=w623, y=w622) -> (x+y=w621:u16)
                        n253 = case shown="False" w628 {
                          tunnel: w626 -> [w636 w640]
                          tunnel: w621 -> [w635 w639]
                          tunnel: [w637 w638] -> w627
                          frame False {
                            n254 = Add(x=w636, y=w635) -> (x+y=w637:u16)
                          }
                          frame True {
                            n255 = Subtract(x=w640, y=w639) -> (x-y=w638:u16)
                          }
                        }
                      }
                    }
                  }
                }
                n256 = Add(x="BD 1 Frequency 2", y=i64 0 ("f")) -> (x+y=w595:u64)
                "BD1 Frequency Out 2" <- w595
              }
              frame 3 {
                # "Fluorescence period"
              }
            }
            n257 = feedback-in #16(w250) -> ()
            n258 = feedback #16(w250) -> (w249:u16)
            n259 = Select(t=w252, s="Interlace ON/OFF", f="Interlace Off Parameters") -> (s? t:f=w289:u8)
            n260 = Subtract(x=w250, y=w249) -> (x-y=w248:u16)
            n261 = Subtract "The error"(x=w248, y=w247) -> (x-y=w225:u16)
            n262 = case shown="1, Default" w289 {
              tunnel: ["DIO count 1 (ticks)" "DIO count 2 (ticks)" "DIO count 3 (ticks)"] -> w246
              frame 1, Default {
              }
              frame 2 {
              }
              frame 3 {
              }
            }
            n263 = Number To Boolean Array(number=w225) -> (Boolean array=w226:bool[])
            n264 = Or Array Elements(Boolean array=w226) -> (logical OR=w224:bool)
            n265 = Boolean To (0,1)(Boolean=w224) -> (0, 1=w231:i16)
            n266 = To Unsigned Byte Integer(number=w231) -> (unsigned 8bit integer=w228:u8)
            n267 = feedback #17(u8 0) -> (w229:u8)
            n268 = Add(x=w228, y=w229) -> (x+y=w227:u8)
            "DIO Late Counter" <- w227
            n269 = feedback-in #17(w227) -> ()
            n270 = Subtract(x=w246, y=w225) -> (x-y=w245:u16)
            n271 = Split Number(x=w286) -> (hi(x)=w285:u32, lo(x)=w284:u32)
            n272 = Split Number(x=w275) -> (hi(x)=w280:u32, lo(x)=w279:u32)
            n273 = Boolean To (0,1)(Boolean="+ phase (DIO)") -> (0, 1=w242:i16)
            n274 = Split Number(x=w285) -> (lo(x)=w283:u16)  [unwired: 1 out]
            n275 = Split Number(x=w284) -> (hi(x)=w282:u16, lo(x)=w281:u16)
            n276 = Split Number(x=w280) -> (lo(x)=w278:u16)  [unwired: 1 out]
            n277 = Split Number(x=w279) -> (hi(x)=w277:u16, lo(x)=w276:u16)
            n278 = Split Number(x=w235) -> (hi(x)=w237:u8, lo(x)=w236:u8)
            n279 = Split Number(x=w232) -> (hi(x)=w234:u8, lo(x)=w233:u8)
            n280 = Split Number(x=w283) -> (hi(x)=w274:u8, lo(x)=w273:u8)
            n281 = Split Number(x=w282) -> (hi(x)=w272:u8, lo(x)=w271:u8)
            n282 = Split Number(x=w278) -> (hi(x)=w267:u8, lo(x)=w266:u8)
            n283 = Split Number(x=w281) -> (hi(x)=w270:u8, lo(x)=w269:u8)
            n284 = Split Number(x=w277) -> (hi(x)=w265:u8, lo(x)=w264:u8)
            n285 = Split Number(x=w276) -> (hi(x)=w263:u8, lo(x)=w262:u8)
            n286 = Multiply(x=w242, y="Phase count adjustment (DIO)") -> (x*y=w238:i16)
            n287 = feedback #18(i16 0) -> (w240:i16)
            n288 = Subtract(x=w240, y=w238) -> (x-y=w239:i16)
            "DIO Relative phase" <- w239
            n289 = feedback-in #18(w239) -> ()
            n290 = Add(x=w245, y=w238) -> (x+y=w244:u16)
            n291 = Build Array "BD 1 A Stack"(w237, w236) -> (w259:u8[])
            n292 = Build Array "BD 2 A Stack"(w234, w233) -> (w258:u8[])
            n293 = Build Array "BD 1 nu Stack"(w274, w273, w272, w271, w270, w269) -> (w268:u8[])
            n294 = Build Array "BD 2 nu Stack"(w267, w266, w265, w264, w263, w262) -> (w261:u8[])
            n295 = case shown="2" w216 {
              tunnel: [w329 w332] -> w257
              tunnel: [u8 10 u8 4] -> w260
              tunnel: "Swap F1 and F2" -> [w330 w332]
              frame 2 {
                # "F2"
                n296 = Not(x=w330) -> (.not. x?=w329:bool)
              }
              frame 1, Default {
                # "low chooses F1"
                # "F1"
              }
            }
            n297 = case "If FPGA is controlling (toggling) RF synth" shown="True" w256 {
              tunnel: w268 -> [_ w305]
              tunnel: w261 -> [_ w304]
              tunnel: w260 -> [_ w303]
              tunnel: w259 -> [_ w302]
              tunnel: w258 -> [_ w301]
              frame False {
              }
              frame True {
                # "Write next amp.\n(wait until beginning of next loop iteration to update)"
                n298 = flat-sequence "Update the next F1 and F2 frequency value (the actual frequency won't change until FSK is switched).\nThen load the next amplitude value into buffer, but don't update it until the next cycle." {
                  tunnel: w304 -> [w307]
                  tunnel: w305 -> [w308]
                  tunnel: [w308] -> w300
                  tunnel: [w307] -> w299
                  tunnel: w303 -> [w309]
                  tunnel: w300 -> [w311]
                  tunnel: w299 -> [w310]
                  tunnel: w302 -> [w322]
                  tunnel: w301 -> [w321]
                  frame #0 {
                    # "To possibly send\nthese writes to very\nend of loop (for x and\ny phase adjust)"
                    n299 = call "Wait8"("Count(Ticks)"="Next trap write delay (ticks)") -> ()  [unwired: 1 out]
                  }
                  frame #1 {
                    n300 = for {
                      tunnel: w311 -> [w317] mode=indexing
                      tunnel: w310 -> [w316] mode=indexing
                      tunnel: w309 -> [w314]
                      i -> [w315]
                      # "Write next freq."
                      n301 = To Unsigned Byte Integer(number=w315) -> (unsigned 8bit integer=w312:u8)
                      n302 = Add(x=w314, y=w312) -> (x+y=w313:u8)
                      n303 = call "write to RF synth bd.vi"("Address Byte"=w313, "BD 2 Byte"=w316, "BD 1 Byte"=w317) -> ()
                    }
                  }
                  frame #2 {
                    w318 = TRUE ("Connector1/DIO15")
                    # "send udclk high\n(BD 1 and 2)"
                    n304 = xnode "FPGA I/O Node"("Connector1/DIO30"=w318, "Connector1/DIO29"=w318) -> ()  [unwired: 2 in, 2 out]
                  }
                  frame #3 {
                    w319 = FALSE ("Connector1/DIO15")
                    n305 = xnode "FPGA I/O Node"("Connector1/DIO30"=w319, "Connector1/DIO29"=w319) -> ()  [unwired: 2 in, 2 out]
                  }
                  frame #4 {
                    n306 = for {
                      tunnel: w322 -> [w328] mode=indexing
                      tunnel: w321 -> [w327] mode=indexing
                      tunnel: u8 33 -> [w325]
                      i -> [w326]
                      n307 = To Unsigned Byte Integer(number=w326) -> (unsigned 8bit integer=w323:u8)
                      n308 = Add(x=w325, y=w323) -> (x+y=w324:u8)
                      n309 = call "write to RF synth bd.vi"("Address Byte"=w324, "BD 2 Byte"=w327, "BD 1 Byte"=w328) -> ()
                    }
                  }
                }
              }
            }
          }
        }
      }
    }
  }
  n310 = while "APD 1 Counter" {
    tunnel: w4 -> [_]
    stop <- FALSE stop-if-true
    n311 = flat-sequence {
      frame #0 {
        n312 = xnode "FPGA I/O Method Node"("FPGA I/O In"=refnum<k21> "Connector0/DIO0" ("APD 1 DO"), "Timeout"=-1) -> ()  [unwired: 2 out]
      }
      frame #1 {
        n313 = local read "APD1 int gate"() -> (w651:bool)
        n314 = case shown="True" w651 {
          frame False {
          }
          frame True {
            n315 = local read "APD1 out state"() -> (w652:bool)
            n316 = case shown="True" w652 {
              frame False {
                n317 = local read "APD 1 Counts 0"() -> (w654:u32)
                n318 = Increment(x=w654) -> (x+1=→"APD 1 Counts 0":u32)
              }
              frame True {
                n319 = local read "APD 1 Counts 1"() -> (w656:u32)
                n320 = Increment(x=w656) -> (x+1=→"APD 1 Counts 1":u32)
              }
            }
          }
        }
      }
    }
  }
  n321 = while "APD 2 Counter" {
    tunnel: w4 -> [_]
    stop <- FALSE stop-if-true
    n322 = flat-sequence {
      frame #0 {
        n323 = xnode "FPGA I/O Method Node"("FPGA I/O In"=refnum<k21> "Connector0/DIO1" ("APD 2 DO"), "Timeout"=-1) -> ()  [unwired: 2 out]
      }
      frame #1 {
        n324 = local read "APD2 int gate"() -> (w660:bool)
        n325 = case shown="True" w660 {
          frame False {
          }
          frame True {
            n326 = local read "APD2 out state"() -> (w661:bool)
            n327 = case shown="False" w661 {
              frame False {
                n328 = local read "APD 2 Counts 0"() -> (w663:u32)
                n329 = Increment(x=w663) -> (x+1=→"APD 2 Counts 0":u32)
              }
              frame True {
                n330 = local read "APD 2 Counts 1"() -> (w665:u32)
                n331 = Increment(x=w665) -> (x+1=→"APD 2 Counts 1":u32)
              }
            }
          }
        }
      }
    }
  }
  n332 = while "APD 2 Gating" {
    shift-right: [w669] -> _
    shift-left: w4 -> [w674]
    shift-right: [w668] -> _
    shift-left: w7 -> [w666]
    stop <- FALSE stop-if-true
    n333 = flat-sequence {
      tunnel: w674 -> [w677]
      tunnel: [w678] -> w672
      tunnel: [w677] -> w670
      tunnel: [w676] -> w667
      tunnel: w666 -> [w676]
      tunnel: [w681] -> w673
      tunnel: w672 -> [w681]
      tunnel: [w680] -> w671
      tunnel: w670 -> [w680]
      tunnel: w667 -> [w679]
      tunnel: [w703] -> w669
      tunnel: w673 -> [w713]
      tunnel: w671 -> [w711]
      tunnel: [w682] -> w668
      frame #0 {
        n334 = call "Loop Timer8"("Count(Ticks)"=w677) -> ("Tick Count(Ticks)"=w678:u16)
      }
      frame #1 {
        # "Signal maybe then sent through \na transistor before APD"
        n335 = xnode "FPGA I/O Node"("Connector0/DIO8"=w679, "Connector0/DIO9"=w679, "Connector0/DIO10"=w679, "Connector0/DIO11"=w679) -> ()  [unwired: 4 in, 4 out]
        "APD2 int gate" <- w679
      }
      frame #2 {
        n336 = local read "APD Gate ON Count"() -> (w696:u16)
        n337 = local read "APD Gate OFF Count"() -> (w695:u16)
        n338 = feedback #19(TRUE) -> (w708:bool)
        n339 = feedback-in #20(w713) -> ()
        n340 = feedback #20(w713) -> (w697:u16)
        n341 = Not(x=w708) -> (.not. x?=w706:bool)
        n342 = feedback-in #19(w706) -> ()
        n343 = Subtract(x=w713, y=w697) -> (x-y=w712:u16)
        n344 = Select(t=w696, s=w706, f=w695) -> (s? t:f=w710:u16)
        n345 = Subtract(x=w712, y=w711) -> (x-y=w688:u16)
        n346 = Subtract(x=w710, y=w688) -> (x-y=w702:u16)
        n347 = Number To Boolean Array(number=w688) -> (Boolean array=w687:bool[])
        n348 = Or Array Elements(Boolean array=w687) -> (logical OR=w686:bool)
        n349 = Boolean To (0,1)(Boolean="+ phase (APD 2 Gate)") -> (0, 1=w700:i16)
        n350 = Multiply(x=w700, y="Phase count adjustment (APD 2 Gate)") -> (x*y=w698:i16)
        n351 = Boolean To (0,1)(Boolean=w686) -> (0, 1=w693:i16)
        n352 = Add(x=w702, y=w698) -> (x+y=w703:u16)
        n353 = To Unsigned Byte Integer(number=w693) -> (unsigned 8bit integer=w690:u8)
        n354 = feedback #21(i16 0) -> (w705:i16)
        n355 = Subtract(x=w705, y=w698) -> (x-y=w704:i16)
        "APD 2 Gate Relative Phase" <- w704
        n356 = feedback-in #21(w704) -> ()
        n357 = feedback #22(u8 0) -> (w691:u8)
        n358 = Add(x=w690, y=w691) -> (x+y=w689:u8)
        "APD 2 Gate Late Counter" <- w689
        n359 = feedback-in #22(w689) -> ()
        n360 = local read "APD Gate Operating Mode"() -> (w694:u8)
        n361 = case shown="2" w694 {
          tunnel: [TRUE FALSE w716] -> w683
          tunnel: w708 -> [_ _ w716]
          frame 0, Default {
          }
          frame 1 {
          }
          frame 2 {
          }
        }
        n362 = local read "Invert APD Gate"() -> (w685:bool)
        n363 = Not(x=w683) -> (.not. x?=w684:bool)
        n364 = Select(t=w684, s=w685, f=w683) -> (s? t:f=w682:bool)
      }
    }
  }
  n365 = while "532 nm green fluorescent laser interlacing (DO to IA 532 nm AOM ME amp)." {
    shift-right: [w720] -> _
    shift-left: w4 -> [w725]
    shift-right: [w719] -> _
    shift-left: w5 -> [w717]
    stop <- FALSE stop-if-true
    n366 = flat-sequence {
      tunnel: w725 -> [w728]
      tunnel: [w729] -> w723
      tunnel: [w728] -> w721
      tunnel: [w727] -> w718
      tunnel: w717 -> [w727]
      tunnel: [w732] -> w724
      tunnel: w723 -> [w732]
      tunnel: [w731] -> w722
      tunnel: w721 -> [w731]
      tunnel: w718 -> [w730]
      tunnel: [w741] -> w720
      tunnel: w724 -> [w761]
      tunnel: w722 -> [w758]
      tunnel: [w750] -> w719
      frame #0 {
        n367 = call "Loop Timer4"("Count(Ticks)"=w728) -> ("Tick Count(Ticks)"=w729:u16)
      }
      frame #1 {
        n368 = xnode "FPGA I/O Node"("Connector1/DIO34"=w730, "Connector1/DIO38"=w730, "Connector1/DIO39"=w730) -> ()  [unwired: 3 in, 3 out]
      }
      frame #2 {
        n369 = feedback-in #23(w761) -> ()
        n370 = feedback #23(w761) -> (w760:u16)
        n371 = Subtract(x=w761, y=w760) -> (x-y=w759:u16)
        n372 = Subtract(x=w759, y=w758) -> (x-y=w734:u16)
        n373 = Number To Boolean Array(number=w734) -> (Boolean array=w735:bool[])
        n374 = Or Array Elements(Boolean array=w735) -> (logical OR=w733:bool)
        n375 = Boolean To (0,1)(Boolean="+ phase (GI)") -> (0, 1=w746:i16)
        n376 = Multiply(x=w746, y="Phase count adjustment (GI)") -> (x*y=w743:i16)
        n377 = Boolean To (0,1)(Boolean=w733) -> (0, 1=w740:i16)
        n378 = To Unsigned Byte Integer(number=w740) -> (unsigned 8bit integer=w737:u8)
        n379 = feedback #24(i16 0) -> (w744:i16)
        n380 = feedback #25(u8 0) -> (w738:u8)
        n381 = Add(x=w737, y=w738) -> (x+y=w736:u8)
        "GI Late Counter" <- w736
        n382 = feedback-in #25(w736) -> ()
        n383 = Subtract(x=w744, y=w743) -> (x-y=w742:i16)
        "GI Relative phase" <- w742
        n384 = feedback-in #24(w742) -> ()
        n385 = feedback #26(TRUE) -> (w753:bool)
        n386 = case shown="2" "Operating Mode" {
          tunnel: [TRUE FALSE w767] -> w750
          tunnel: w753 -> [_ _ w764]
          frame 0, Default {
          }
          frame 1 {
          }
          frame 2 {
            n387 = Not(x=w764) -> (.not. x?=w766:bool)
            n388 = Select(t=w766, s="Invert GI", f=w764) -> (s? t:f=w767:bool)
          }
        }
        n389 = Not(x=w753) -> (.not. x?=w749:bool)
        n390 = Select(t="Green interlace ON count", s=w749, f="Green interlace OFF count") -> (s? t:f=w755:u16)
        n391 = Subtract(x=w755, y=w734) -> (x-y=w747:u16)
        n392 = Add(x=w747, y=w743) -> (x+y=w741:u16)
        n393 = feedback-in #26(w749) -> ()
      }
    }
  }
  n394 = while "Green and red fluorescent laser interlacing (Current AO to IA 532 nm AOM ME amp)." {
    shift-right: [w776] -> _
    shift-left: w4 -> [w779]
    shift-right: [w773] -> _
    shift-left: w6 -> [w771]
    shift-right: [w770] -> _
    shift-left: w6 -> [w769]
    stop <- FALSE stop-if-true
    n395 = flat-sequence {
      tunnel: w779 -> [w783]
      tunnel: [w784] -> w778
      tunnel: [w783] -> w777
      tunnel: [w782] -> w772
      tunnel: w771 -> [w782]
      tunnel: w769 -> [w781]
      tunnel: [w781] -> w768
      tunnel: [w788] -> w775
      tunnel: w778 -> [w788]
      tunnel: [w787] -> w774
      tunnel: w777 -> [w787]
      tunnel: w772 -> [w786]
      tunnel: w768 -> [w785]
      tunnel: [w801] -> w776
      tunnel: [w817] -> w773
      tunnel: w775 -> [w828]
      tunnel: w774 -> [w825]
      tunnel: [w791] -> w770
      frame #0 {
        n396 = call "Loop Timer10"("Count(Ticks)"=w783) -> ("Tick Count(Ticks)"=w784:u16)
      }
      frame #1 {
        n397 = xnode "FPGA I/O Node"("Chassis2/Mod1/AO0"=w786, "Chassis2/Mod1/AO1"=w785) -> ()  [unwired: 2 in, 2 out]
      }
      frame #2 {
        # "Design note:\n\nThese two laser controls are in the same loop\nbecause the expansion current AI cannot separately\ntime the outputs fast enough for us.  Apparently\nit is because of communication time between the\nexpansion card and the fpga.\n\nSo the two analog control signals have the same timing\nand profile, but independent amplitudes to independently\ncontrol the intensity and feedback for each laser."
        n398 = feedback #27(TRUE) -> (w789:bool)
        n399 = Not(x=w789) -> (.not. x?=w790:bool)
        n400 = feedback-in #27(w790) -> ()
        n401 = Subtract(x="Green interlace OFF count 2", y="Green int current ON count adj") -> (x-y=w810:u16)
        n402 = disable-structure shown="Disabled" {
          disable-tunnel: [w832 _] -> w791
          disable-tunnel: w789 -> [w829 _]
          frame Disabled {
            n403 = case shown="2" "RI Operating Mode 2" {
              tunnel: [TRUE FALSE w844] -> w830
              tunnel: w829 -> [_ _ w841]
              frame 0, Default {
              }
              frame 1 {
              }
              frame 2 {
                n404 = Not(x=w841) -> (.not. x?=w843:bool)
                n405 = Select(t=w843, s="Invert RI 2", f=w841) -> (s? t:f=w844:bool)
              }
            }
            n406 = And(x=w830, y="Red FB On/Off") -> (x .and. y?=w838:bool)
            n407 = case shown="True" w838 {
              tunnel: "RI Current Out" -> [w845 _]
              tunnel: [w845 w854] -> w834
              frame False {
              }
              frame True {
                n408 = local read "Red FB Intensity"() -> (w850:i16)
                n409 = Bundle("P4"="P4", "I4"="I4", "D4"="D4") -> (w846:cluster{"P4":i16, "I4":i16, "D4":i16})  [unwired: 1 in]
                n410 = call "Slower PID.vi"("process variable"=w850, "reset?"="Red FB Reset", "setpoint"="Red FB Setpoint", "PID gains (x 2^8)"=w846, "output range"=cluster{"output high":i16, "output low":i16} {"output high"=32767, "output low"=-32768} ("Green FB output range")) -> ("output"=w857:i16)  [unwired: 10 out]
                n411 = To Long Integer(number=w857) -> (32bit integer=w851:i32)
                n412 = Add(x=w851, y=32768) -> (x+y=w853:i32)
                n413 = To Unsigned Word Integer(number=w853) -> (unsigned 16bit integer=w854:u16)
              }
            }
            n414 = Boolean To (0,1)(Boolean=w830) -> (0, 1=w833:i16)
            n415 = To Unsigned Word Integer(number=w833) -> (unsigned 16bit integer=w835:u16)
            n416 = Multiply(x=w835, y=w834) -> (x*y=w832:u16)
          }
          frame Enabled {
          }
        }
        n417 = feedback-in #28(w828) -> ()
        n418 = feedback #28(w828) -> (w827:u16)
        n419 = Add(x="Green int current ON count adj", y="Green interlace ON count 2") -> (x+y=w811:u16)
        n420 = Subtract(x=w828, y=w827) -> (x-y=w826:u16)
        n421 = Select(t=w811, s=w790, f=w810) -> (s? t:f=w822:u16)
        n422 = Subtract(x=w826, y=w825) -> (x-y=w794:u16)
        n423 = Subtract(x=w822, y=w794) -> (x-y=w805:u16)
        n424 = case shown="2" "Operating Mode 2" {
          tunnel: [TRUE FALSE w878] -> w792
          tunnel: w789 -> [_ _ w875]
          frame 0, Default {
          }
          frame 1 {
          }
          frame 2 {
            n425 = Not(x=w875) -> (.not. x?=w877:bool)
            n426 = Select(t=w877, s="Invert GI 2", f=w875) -> (s? t:f=w878:bool)
          }
        }
        n427 = Number To Boolean Array(number=w794) -> (Boolean array=w795:bool[])
        n428 = Boolean To (0,1)(Boolean="+ phase (GI) 2") -> (0, 1=w807:i16)
        n429 = Or Array Elements(Boolean array=w795) -> (logical OR=w793:bool)
        n430 = Boolean To (0,1)(Boolean=w793) -> (0, 1=w800:i16)
        n431 = Multiply(x=w807, y="Phase count adjustment (GI) 2") -> (x*y=w803:i16)
        n432 = To Unsigned Byte Integer(number=w800) -> (unsigned 8bit integer=w796:u8)
        n433 = Add(x=w805, y=w803) -> (x+y=w801:u16)
        n434 = feedback #29(u8 0) -> (w798:u8)
        n435 = Add(x=w796, y=w798) -> (x+y=w797:u8)
        "GI Late Counter 2" <- w797
        n436 = feedback-in #29(w797) -> ()
        n437 = feedback #30(i16 0) -> (w804:i16)
        n438 = Subtract(x=w804, y=w803) -> (x-y=w802:i16)
        "GI Relative phase 2" <- w802
        n439 = feedback-in #30(w802) -> ()
        n440 = And(x=w792, y="Green FB On/Off") -> (x .and. y?=w812:bool)
        n441 = case shown="False" w812 {
          tunnel: "Current Out" -> [w859 _]
          tunnel: [w859 w868] -> w816
          frame False {
          }
          frame True {
            n442 = local read "Green FB Sum"() -> (w864:i16)
            n443 = Bundle("P3"="P3", "I3"="I3", "D3"="D3") -> (w860:cluster{"P3":i16, "I3":i16, "D3":i16})  [unwired: 1 in]
            n444 = call "Slower PID.vi"("process variable"=w864, "reset?"="Green FB Reset", "setpoint"="Green FB Setpoint", "PID gains (x 2^8)"=w860, "output range"=cluster{"output high":i16, "output low":i16} {"output high"=32767, "output low"=-32768} ("Green FB output range")) -> ("output"=w871:i16)  [unwired: 10 out]
            n445 = To Long Integer(number=w871) -> (32bit integer=w865:i32)
            n446 = Add(x=w865, y=32768) -> (x+y=w867:i32)
            n447 = To Unsigned Word Integer(number=w867) -> (unsigned 16bit integer=w868:u16)
          }
        }
        n448 = Boolean To (0,1)(Boolean=w792) -> (0, 1=w818:i16)
        n449 = To Unsigned Word Integer(number=w818) -> (unsigned 16bit integer=w815:u16)
        n450 = Multiply(x=w815, y=w816) -> (x*y=w817:u16)
      }
    }
  }
  n451 = while "APD 1 Gating" {
    shift-right: [w882] -> _
    shift-left: w4 -> [w887]
    shift-right: [w881] -> _
    shift-left: w7 -> [w879]
    stop <- FALSE stop-if-true
    n452 = flat-sequence {
      tunnel: w887 -> [w890]
      tunnel: [w891] -> w885
      tunnel: [w890] -> w883
      tunnel: [w889] -> w880
      tunnel: w879 -> [w889]
      tunnel: [w894] -> w886
      tunnel: w885 -> [w894]
      tunnel: [w893] -> w884
      tunnel: w883 -> [w893]
      tunnel: w880 -> [w892]
      tunnel: [w912] -> w882
      tunnel: w886 -> [w926]
      tunnel: w884 -> [w923]
      tunnel: [w895] -> w881
      frame #0 {
        n453 = call "Loop Timer7"("Count(Ticks)"=w890) -> ("Tick Count(Ticks)"=w891:u16)
      }
      frame #1 {
        # "Signal maybe then sent through \na transistor before APD"
        n454 = xnode "FPGA I/O Node"("Connector0/DIO4"=w892, "Connector0/DIO5"=w892, "Connector0/DIO6"=w892, "Connector0/DIO7"=w892) -> ()  [unwired: 4 in, 4 out]
        "APD1 int gate" <- w892
      }
      frame #2 {
        n455 = feedback #31(TRUE) -> (w918:bool)
        n456 = feedback-in #32(w926) -> ()
        n457 = feedback #32(w926) -> (w925:u16)
        n458 = Not(x=w918) -> (.not. x?=w915:bool)
        n459 = feedback-in #31(w915) -> ()
        n460 = Subtract(x=w926, y=w925) -> (x-y=w924:u16)
        n461 = Select(t="APD Gate ON Count", s=w915, f="APD Gate OFF Count") -> (s? t:f=w920:u16)
        n462 = Subtract(x=w924, y=w923) -> (x-y=w900:u16)
        n463 = Subtract(x=w920, y=w900) -> (x-y=w911:u16)
        n464 = Number To Boolean Array(number=w900) -> (Boolean array=w901:bool[])
        n465 = Or Array Elements(Boolean array=w901) -> (logical OR=w899:bool)
        n466 = Boolean To (0,1)(Boolean="+ phase (APD 1 Gate)") -> (0, 1=w909:i16)
        n467 = Boolean To (0,1)(Boolean=w899) -> (0, 1=w906:i16)
        n468 = Multiply(x=w909, y="Phase count adjustment (APD 1 Gate)") -> (x*y=w907:i16)
        n469 = To Unsigned Byte Integer(number=w906) -> (unsigned 8bit integer=w903:u8)
        n470 = Add(x=w911, y=w907) -> (x+y=w912:u16)
        n471 = feedback #33(i16 0) -> (w914:i16)
        n472 = Subtract(x=w914, y=w907) -> (x-y=w913:i16)
        "APD 1 Gate Relative Phase" <- w913
        n473 = feedback-in #33(w913) -> ()
        n474 = feedback #34(u8 0) -> (w904:u8)
        n475 = Add(x=w903, y=w904) -> (x+y=w902:u8)
        "APD 1 Gate Late Counter" <- w902
        n476 = feedback-in #34(w902) -> ()
        n477 = case shown="2" "APD Gate Operating Mode" {
          tunnel: [TRUE FALSE w929] -> w896
          tunnel: w918 -> [_ _ w929]
          frame 0, Default {
          }
          frame 1 {
          }
          frame 2 {
          }
        }
        n478 = Not(x=w896) -> (.not. x?=w897:bool)
        n479 = Select(t=w897, s="Invert APD Gate", f=w896) -> (s? t:f=w895:bool)
      }
    }
  }
  n480 = while "MCL stage control" {
    shift-right: [w942] -> _
    shift-left: w4 -> [w945]
    shift-right: [w935] -> _
    shift-left: w12 -> [w932]
    shift-right: [w934] -> _
    shift-left: w11 -> [w930]
    stop <- FALSE stop-if-true
    n481 = flat-sequence {
      tunnel: w945 -> [w949]
      tunnel: [w950] -> w941
      tunnel: [w949] -> w939
      tunnel: [w948] -> w933
      tunnel: w932 -> [w948]
      tunnel: [w947] -> w931
      tunnel: w930 -> [w947]
      tunnel: w941 -> [w954]
      tunnel: [w954] -> w940
      tunnel: w939 -> [w953]
      tunnel: [w953] -> w938
      tunnel: w933 -> [w952]
      tunnel: w931 -> [w951]
      tunnel: w940 -> [w962]
      tunnel: w938 -> [w961]
      tunnel: [w962] -> w944
      tunnel: [w961] -> w943
      tunnel: [w960] -> w937
      tunnel: [w959] -> w936
      tunnel: [w1034] -> w942
      tunnel: w944 -> [w1041]
      tunnel: w943 -> [w1038]
      tunnel: w937 -> [w1036]
      tunnel: w936 -> [w1035]
      tunnel: [w1036] -> w935
      tunnel: [w1035] -> w934
      frame #0 {
        n482 = call "Loop Timer5"("Count(Ticks)"=w949) -> ("Tick Count(Ticks)"=w950:u32)
      }
      frame #1 {
        n483 = xnode "FPGA I/O Node"("Connector0/AO1"=w952, "Connector0/AO2"=w951) -> ()  [unwired: 2 in, 2 out]
      }
      frame #2 {
        n484 = local read "Scanning MCL"() -> (w974:bool)
        n485 = Or(x=w974, y="Start scan (MCL)") -> (x .or. y?=w969:bool)
        n486 = Not(x="Abort scan (MCL)") -> (.not. x?=w967:bool)
        n487 = And(x=w967, y=w969) -> (x .and. y?=w966:bool)
        n488 = case "Raster scan" shown="True" w966 {
          tunnel: [w975 w1018] -> w971
          tunnel: "Start scan (MCL)" -> [_ w1003]
          tunnel: [w975 w979] -> w955
          frame False {
            w975 = i16 0
            n489 = local write "Scanning MCL"(FALSE ("scanning")) -> ()
          }
          frame True {
            w989 = i16 0
            w988 = u64 0
            # "scan incr."
            # "freq. incr. mult."
            # "count steps"
            # "count number of cycles"
            n490 = feedback #35(w988) -> (w1015:u64)
            n491 = Select(t=w988, s=w1003, f=w1015) -> (s? t:f=w1017:u64)
            n492 = Increment(x=w1017) -> (x+1=w1014:u64)
            n493 = Greater?(x="Cycles per step (MCL)", y=w1014) -> (0:w998:bool)
            n494 = Select(t=w1014, s=w998, f=w988) -> (s? t:f=w1013:u64)
            n495 = feedback-in #35(w1013) -> ()
            n496 = feedback #36(w988) -> (w1012:u64)
            n497 = Select(t=w988, s=w1003, f=w1012) -> (s? t:f=w1007:u64)
            n498 = Increment(x=w1007) -> (x+1=w1011:u64)
            n499 = Add(x="Scan steps (MCL)", y="Scan steps (MCL)") -> (x+y=w1010:u64)
            n500 = Select(t=w1007, s=w998, f=w1011) -> (s? t:f=w993:u64)
            n501 = Greater?(x=w1010, y=w993) -> (0:w992:bool)
            n502 = Select(t=w993, s=w992, f=w988) -> (s? t:f=w1008:u64)
            n503 = feedback-in #36(w1008) -> ()
            n504 = Equal?(x="Scan steps (MCL)", y=w993) -> (x = y?=w997:bool)
            n505 = Greater?(x="Scan steps (MCL)", y=w1007) -> (0:w1006:bool)
            n506 = feedback #37(w989) -> (w1009:i16)
            n507 = Select(t=w989, s=w1003, f=w1009) -> (s? t:f=w995:i16)
            n508 = Increment(x=w995) -> (x+1=w1005:i16)
            n509 = Decrement(x=w995) -> (x-1=w1004:i16)
            n510 = Select(t=w1005, s=w1006, f=w1004) -> (s? t:f=w996:i16)
            n511 = Select(t=w995, s=w997, f=w996) -> (s? t:f=w994:i16)
            n512 = Select(t=w995, s=w998, f=w994) -> (s? t:f=w990:i16)
            n513 = Select(t=w990, s=w992, f=w989) -> (s? t:f=w991:i16)
            n514 = feedback-in #37(w991) -> ()
            n515 = feedback #38(w988) -> (w1002:u64)
            n516 = Select(t=w988, s=w1003, f=w1002) -> (s? t:f=w977:u64)
            n517 = Increment(x=w977) -> (x+1=w999:u64)
            n518 = Select(t=w977, s=w992, f=w999) -> (s? t:f=w978:u64)
            n519 = Greater?(x="Number of scans (MCL)", y=w978) -> (0:w985:bool)
            n520 = Multiply(x="Scan freq.  increment (MCL)", y=w995) -> (x*y=w1018:i16)
            n521 = Select(t=TRUE, s="Cont. Scan (MCL)", f=w985) -> (s? t:f=w984:bool)
            "Scanning MCL" <- w984
            n522 = Select(t=w978, s=w984, f=w988) -> (s? t:f=w1000:u64)
            n523 = feedback-in #38(w1000) -> ()
            n524 = Increment(x=w978) -> (x+1=→"Scan I (MCL)":u64)
            n525 = To Word Integer(number=w977) -> (16bit integer=w980:i16)
            n526 = Multiply(x=w980, y="Scan freq.  increment (MCL)") -> (x*y=w979:i16)
          }
        }
        n527 = Select(t=w955, s="1D or 2D Scan?", f=i16 0) -> (s? t:f=w956:i16)
        n528 = Select(t=w956, s="MCL Scan Axis", f=w971) -> (s? t:f=w970:i16)
        n529 = Select(t=w971, s="MCL Scan Axis", f=w956) -> (s? t:f=w972:i16)
        n530 = Add(x=w970, y="AO2") -> (x+y=w959:i16)
        n531 = Add(x="AO1", y=w972) -> (x+y=w960:i16)
      }
      frame #3 {
        n532 = feedback-in #39(w1041) -> ()
        n533 = feedback #39(w1041) -> (w1040:u32)
        n534 = Boolean To (0,1)(Boolean="+ phase (MCL)") -> (0, 1=w1032:i16)
        n535 = Subtract(x=w1041, y=w1040) -> (x-y=w1039:u32)
        n536 = Multiply(x=w1032, y="Phase count adjustment (MCL)") -> (x*y=w1028:i16)
        n537 = Subtract(x=w1039, y=w1038) -> (x-y=w1020:u32)
        n538 = Subtract(x="MCL count", y=w1020) -> (x-y=w1030:u32)
        n539 = feedback #40(i16 0) -> (w1029:i16)
        n540 = Subtract(x=w1029, y=w1028) -> (x-y=w1027:i16)
        "MCL Relative Phase" <- w1027
        n541 = feedback-in #40(w1027) -> ()
        n542 = Number To Boolean Array(number=w1020) -> (Boolean array=w1021:bool[])
        n543 = Or Array Elements(Boolean array=w1021) -> (logical OR=w1019:bool)
        n544 = Boolean To (0,1)(Boolean=w1019) -> (0, 1=w1026:i16)
        n545 = Add(x=w1030, y=w1028) -> (x+y=w1034:u32)
        n546 = To Unsigned Byte Integer(number=w1026) -> (unsigned 8bit integer=w1023:u8)
        n547 = feedback #41(u8 0) -> (w1024:u8)
        n548 = Add(x=w1023, y=w1024) -> (x+y=w1022:u8)
        "MCL Late Counter" <- w1022
        n549 = feedback-in #41(w1022) -> ()
      }
    }
  }
  n550 = while "Control APD data integration - stream to host" {
    shift-right: [w1046] -> _
    shift-left: w8 -> [w1051]
    stop <- FALSE stop-if-true
    n551 = flat-sequence {
      tunnel: w1051 -> [w1053]
      tunnel: [w1054] -> w1049
      tunnel: [w1053] -> w1047
      tunnel: [w1064] -> w1050
      tunnel: w1049 -> [w1064]
      tunnel: [w1063] -> w1048
      tunnel: w1047 -> [w1063]
      tunnel: [w1062] -> w1045
      tunnel: [w1061] -> w1044
      tunnel: [w1055] -> w1043
      tunnel: [w1106] -> w1046
      tunnel: w1050 -> [w1116]
      tunnel: w1048 -> [w1113]
      tunnel: w1045 -> [w1099]
      tunnel: w1044 -> [w1098]
      tunnel: w1043 -> [w1086]
      frame #0 {
        n552 = call "Loop Timer6"("Count(Ticks)"=w1053) -> ("Tick Count(Ticks)"=w1054:u32)
      }
      frame #1 {
        n553 = flat-sequence {
          tunnel: [w1066] -> w1060
          tunnel: w1060 -> [w1069]
          tunnel: [w1073] -> w1059
          tunnel: [w1072] -> w1058
          tunnel: [w1069] -> w1057
          tunnel: [w1068] -> w1056
          tunnel: [w1080] -> w1061
          tunnel: [w1081] -> w1062
          tunnel: w1059 -> [w1081]
          tunnel: w1058 -> [w1080]
          tunnel: w1057 -> [w1079]
          tunnel: w1056 -> [w1078]
          tunnel: [w1078] -> w1055
          frame #0 {
            # "use separate variable so each APD won't\nhave to wait to read"
            n554 = feedback #42(FALSE) -> (w1065:bool)
            "APD1 out state" <- w1065
            "APD2 out state" <- w1065
            "APD3 out state" <- w1065
            n555 = Not(x=w1065) -> (.not. x?=w1066:bool)
            n556 = feedback-in #42(w1066) -> ()
          }
          frame #1 {
            n557 = local read "APD 3 Counts 1"() -> (w1071:u32)
            n558 = local read "APD 3 Counts 0"() -> (w1070:u32)
            n559 = local read "APD 1 Counts 1"() -> (w1077:u32)
            n560 = local read "APD 1 Counts 0"() -> (w1076:u32)
            n561 = local read "APD 2 Counts 1"() -> (w1075:u32)
            n562 = local read "APD 2 Counts 0"() -> (w1074:u32)
            n563 = Select(t=w1071, s=w1069, f=w1070) -> (s? t:f=w1068:u32)
            n564 = Select(t=w1077, s=w1069, f=w1076) -> (s? t:f=w1073:u32)
            n565 = Select(t=w1075, s=w1069, f=w1074) -> (s? t:f=w1072:u32)
          }
          frame #2 {
            n566 = case shown="False" w1079 {
              frame False {
                w1082 = u32 0 ("APD 1 Counts 0")
                n567 = local write "APD 1 Counts 0"(w1082) -> ()
                n568 = local write "APD 2 Counts 0"(w1082) -> ()
                n569 = local write "APD 3 Counts 0"(w1082) -> ()
              }
              frame True {
                w1083 = u32 0 ("APD 1 Counts 1")
                n570 = local write "APD 1 Counts 1"(w1083) -> ()
                n571 = local write "APD 2 Counts 1"(w1083) -> ()
                n572 = local write "APD 3 Counts 1"(w1083) -> ()
              }
            }
          }
        }
      }
      frame #2 {
        n573 = feedback-in #43(w1116) -> ()
        n574 = feedback #43(w1116) -> (w1115:u32)
        n575 = Subtract(x=w1116, y=w1115) -> (x-y=w1114:u32)
        n576 = Subtract(x=w1114, y=w1113) -> (x-y=w1091:u32)
        n577 = case shown="True" "APD to FIFO" {
          tunnel: w1099 -> [_ w1121]
          tunnel: w1098 -> [_ w1119]
          tunnel: w1086 -> [_ w1117]
          frame False {
          }
          frame True {
            n578 = flat-sequence {
              tunnel: 0 ("Timeout") -> [w1123]
              tunnel: w1121 -> [w1124]
              tunnel: [w1123] -> w1120
              tunnel: w1120 -> [w1125]
              tunnel: w1119 -> [w1126]
              tunnel: [w1125] -> w1118
              tunnel: w1118 -> [w1128]
              tunnel: w1117 -> [w1127]
              frame #0 {
                n579 = xnode ("FIFO Write")("Element"=w1124, "Timeout"=w1123) -> ()  [unwired: 1 in, 2 out]
              }
              frame #1 {
                n580 = xnode ("FIFO Write")("Element"=w1126, "Timeout"=w1125) -> ()  [unwired: 1 in, 2 out]
              }
              frame #2 {
                n581 = xnode ("FIFO Write")("Element"=w1127, "Timeout"=w1128) -> ()  [unwired: 1 in, 2 out]
              }
            }
          }
        }
        n582 = Subtract(x="APD Acq Rate Count", y=w1091) -> (x-y=w1107:u32)
        n583 = Number To Boolean Array(number=w1091) -> (Boolean array=w1092:bool[])
        n584 = Or Array Elements(Boolean array=w1092) -> (logical OR=w1090:bool)
        n585 = Boolean To (0,1)(Boolean=w1090) -> (0, 1=w1097:i16)
        n586 = To Unsigned Byte Integer(number=w1097) -> (unsigned 8bit integer=w1094:u8)
        n587 = feedback #44(u8 0) -> (w1095:u8)
        n588 = Add(x=w1094, y=w1095) -> (x+y=w1093:u8)
        "APD Acq Late Counter" <- w1093
        n589 = feedback-in #44(w1093) -> ()
        n590 = Boolean To (0,1)(Boolean="+ phase (APD Acq)") -> (0, 1=w1103:i16)
        n591 = Multiply(x=w1103, y="Phase Count Adjustment (APD Acq)") -> (x*y=w1100:i16)
        n592 = Add(x=w1107, y=w1100) -> (x+y=w1106:u32)
        n593 = feedback #45(i16 0) -> (w1105:i16)
        n594 = Subtract(x=w1105, y=w1100) -> (x-y=w1102:i16)
        "APD Acq Relative Phase" <- w1102
        n595 = feedback-in #45(w1102) -> ()
        n596 = To Word Integer(number=w1099) -> (16bit integer=w1108:i16)
        n597 = To Word Integer(number=w1086) -> (16bit integer=w1087:i16)
        n598 = To Word Integer(number=w1098) -> (16bit integer=w1109:i16)
        n599 = Multiply(x="APD AO scale factor", y=w1109) -> (x*y=w1088:i16)
        n600 = Multiply(x="APD AO scale factor", y=w1087) -> (x*y=w1084:i16)
        n601 = Multiply(x="APD AO scale factor", y=w1108) -> (x*y=w1089:i16)
        n602 = xnode "FPGA I/O Node"("Connector0/AO6"=w1089, "Connector0/AO7"=w1088, "Connector0/AO5"=w1084) -> ()  [unwired: 3 in, 3 out]
      }
    }
  }
  n603 = while "DAQ AI set 1" {
    shift-right: [w1129] -> _
    shift-left: w4 -> [w1134]
    stop <- FALSE stop-if-true
    n604 = flat-sequence {
      tunnel: w1134 -> [w1144]
      tunnel: [w1145] -> w1132
      tunnel: [w1144] -> w1131
      tunnel: [w1155] -> w1142
      tunnel: [w1154] -> w1141
      tunnel: [w1153] -> w1140
      tunnel: [w1152] -> w1139
      tunnel: [w1151] -> w1138
      tunnel: [w1150] -> w1137
      tunnel: [w1149] -> w1136
      tunnel: [w1148] -> w1135
      tunnel: [w1147] -> w1133
      tunnel: w1132 -> [w1147]
      tunnel: w1131 -> [w1146]
      tunnel: [w1146] -> w1130
      tunnel: [w1185] -> w1129
      tunnel: w1142 -> [w1211]
      tunnel: w1141 -> [w1177]
      tunnel: w1140 -> [w1178]
      tunnel: w1139 -> [w1157]
      tunnel: w1138 -> [w1201]
      tunnel: w1137 -> [w1200]
      tunnel: w1136 -> [w1199]
      tunnel: w1135 -> [w1198]
      tunnel: w1133 -> [w1195]
      tunnel: w1130 -> [w1192]
      frame #0 {
        n605 = call "Loop Timer3"("Count(Ticks)"=w1144) -> ("Tick Count(Ticks)"=w1145:u16)
      }
      frame #1 {
        n606 = xnode "FPGA I/O Node"("Connector1/DIO31"=TRUE ("Connector1/DIO33")) -> ("Connector0/AI0"=w1155:i16, "Connector0/AI1"=w1154:i16, "Connector0/AI2"=w1153:i16, "Connector0/AI3"=w1152:i16, "Connector0/AI4"=w1151:i16, "Connector0/AI5"=w1150:i16, "Connector0/AI6"=w1149:i16, "Connector0/AI7"=w1148:i16)  [unwired: 9 in, 9 out]
      }
      frame #2 {
        w1181 = FALSE ("AI to FIFO")
        # "Adjust phase after data acquired if button pressed"
        n607 = feedback #46(i16 1) -> (w1204:i16)
        n608 = Increment(x=w1204) -> (x+1=w1210:i16)
        n609 = Scale By Power Of 2(n="AI1 X Scale", x=w1177) -> (x*2^n=w1175:i16)
        n610 = Greater?(x=w1210, y="N of AI1 Int Acq Sets") -> (0:w1207:bool)
        n611 = Select(t=i16 1, s=w1207, f=w1210) -> (s? t:f=w1209:i16)
        n612 = feedback-in #46(w1209) -> ()
        n613 = Divide(x=w1175, y=w1157) -> (x/y=w1174:fxp<+/-,16,1>)
        n614 = feedback #47(w1181) -> (w1179:bool)
        n615 = feedback #48(w1181) -> (w1197:bool)
        n616 = case shown="2" w1204 {
          tunnel: w1178 -> [w1234 w1241 _]
          tunnel: ["Set 1" "Set 2" "Set 3"] -> w1202
          tunnel: ["AI to FIFO" w1243 w1248] -> w1196
          tunnel: w1197 -> [_ w1243 w1248]
          tunnel: ["Trap Pos to FIFO" w1242 w1247] -> w1180
          tunnel: w1179 -> [_ w1242 w1247]
          tunnel: w1174 -> [w1233 w1240 _]
          tunnel: [w1232 w1238 FALSE] -> w1161
          tunnel: [w1231 w1239 u64 0 ("BD1 Frequency Out 2")] -> w1160
          frame 1, Default {
            n617 = local read "BD1 Frequency Out 1"() -> (w1231:u64)
            n618 = Compound Arithmetic op=AND("Trap Pos to FIFO", "Set 1", "AI to FIFO") -> (w1232:bool)
            "AI2 Y Sum Set 1" <- w1234
            "AI1 X Set 1" <- w1233
          }
          frame 2 {
            n619 = local read "BD1 Frequency Out 2"() -> (w1239:u64)
            n620 = Compound Arithmetic op=AND(w1242, "Set 2", w1243) -> (w1238:bool)
            "AI2 Y Sum Set 2" <- w1241
            "AI1 X Set 2" <- w1240
          }
          frame 3 {
          }
        }
        n621 = And(x=w1202, y=w1196) -> (x .and. y?=w1203:bool)
        n622 = case shown="True" w1203 {
          tunnel: w1211 -> [_ w1262]
          tunnel: w1177 -> [_ w1261]
          tunnel: w1178 -> [_ w1260]
          tunnel: w1157 -> [_ w1259]
          tunnel: w1201 -> [_ w1258]
          tunnel: w1200 -> [_ w1257]
          tunnel: w1199 -> [_ w1256]
          tunnel: w1198 -> [_ w1255]
          tunnel: 0 ("DMA buffer timeout") -> [_ w1264]
          frame False {
          }
          frame True {
            n623 = Build Array(w1262, w1261, w1260, w1259, w1258, w1257, w1256, w1255) -> (w1263:i16[])
            n624 = for {
              tunnel: w1263 -> [w1266] mode=indexing
              tunnel: w1264 -> [w1267]
              tunnel: [w1265] -> w1253 mode=indexing
              n625 = xnode ("FIFO Write")("Element"=w1266, "Timeout"=w1267) -> ("Timed Out?"=w1265:bool)  [unwired: 1 in, 1 out]
            }
            n626 = Or Array Elements(Boolean array=w1253) -> (logical OR=w1250:bool)
            n627 = Boolean To (0,1)(Boolean=w1250) -> (0, 1=w1252:i16)
            n628 = feedback #49(u16 0) -> (w1251:u16)
            n629 = Add(x=w1252, y=w1251) -> (x+y=w1249:u16)
            "Trap AI FIFO Timeout" <- w1249
            n630 = feedback-in #49(w1249) -> ()
          }
        }
        n631 = feedback-in #47(w1180) -> ()
        n632 = feedback-in #48(w1196) -> ()
        n633 = case shown="True" w1161 {
          tunnel: w1160 -> [_ w1217]
          tunnel: [u8 0 w1214] -> w1159
          frame False {
          }
          frame True {
            n634 = Split Number(x=w1217) -> (hi(x)=w1218:u32, lo(x)=w1219:u32)
            n635 = Split Number(x=w1218) -> (lo(x)=w1220:u16)  [unwired: 1 out]
            n636 = Split Number(x=w1219) -> (hi(x)=w1221:u16, lo(x)=w1222:u16)
            n637 = Build Array "BD 1 nu Stack"(w1220, w1221, w1222) -> (w1216:u16[])
            n638 = for {
              tunnel: w1216 -> [w1229] mode=indexing
              shift-right: [w1225] -> w1214
              shift-left: u8 0 -> [w1226]
              n639 = xnode ("FIFO Method Node")("Element"=w1229, "Timeout"="Trap FIFO Set Timeout") -> ("Timed Out?"=w1228:bool)  [unwired: 1 in, 1 out]
              n640 = Boolean To (0,1)(Boolean=w1228) -> (0, 1=w1227:i16)
              n641 = To Unsigned Byte Integer(number=w1227) -> (unsigned 8bit integer=w1224:u8)
              n642 = Add(x=w1224, y=w1226) -> (x+y=w1225:u8)
            }
          }
        }
        n643 = To Unsigned Word Integer(number=w1159) -> (unsigned 16bit integer=w1158:u16)
        n644 = feedback #50(u16 0) -> (w1172:u16)
        n645 = Add(x=w1158, y=w1172) -> (x+y=w1171:u16)
        "Trap Pos FIFO Timeout" <- w1171
        n646 = feedback-in #50(w1171) -> ()
        n647 = feedback-in #51(w1195) -> ()
        n648 = feedback #51(w1195) -> (w1194:u16)
        n649 = Subtract(x=w1195, y=w1194) -> (x-y=w1193:u16)
        n650 = xnode "FPGA I/O Node"("Connector1/DIO31"=FALSE ("Connector1/DIO34")) -> ()  [unwired: 1 in, 1 out]
        n651 = Subtract(x=w1193, y=w1192) -> (x-y=w1163:u16)
        n652 = Boolean To (0,1)(Boolean="+ phase") -> (0, 1=w1188:i16)
        n653 = Multiply(x=w1188, y="Phase count adjustment") -> (x*y=w1182:i16)
        n654 = Subtract(x="ai count", y=w1163) -> (x-y=w1186:u16)
        n655 = Number To Boolean Array(number=w1163) -> (Boolean array=w1164:bool[])
        n656 = feedback #52(i16 0) -> (w1184:i16)
        n657 = Add(x=w1186, y=w1182) -> (x+y=w1185:u16)
        n658 = Subtract(x=w1184, y=w1182) -> (x-y=w1183:i16)
        "Relative phase" <- w1183
        n659 = feedback-in #52(w1183) -> ()
        n660 = Or Array Elements(Boolean array=w1164) -> (logical OR=w1162:bool)
        n661 = Boolean To (0,1)(Boolean=w1162) -> (0, 1=w1169:i16)
        n662 = To Unsigned Byte Integer(number=w1169) -> (unsigned 8bit integer=w1166:u8)
        n663 = feedback #53(u8 0) -> (w1167:u8)
        n664 = Add(x=w1166, y=w1167) -> (x+y=w1165:u8)
        "AI Late Counter" <- w1165
        n665 = feedback-in #53(w1165) -> ()
      }
    }
  }
  n666 = node-c288(w9) -> ()
  n667 = disable-structure shown="Disabled" {
    disable-tunnel: w4 -> [w1268 _]
    frame Disabled {
      n668 = while "APD 3 Counter" {
        tunnel: w1268 -> [_]
        stop <- FALSE stop-if-true
        n669 = flat-sequence {
          frame #0 {
            n670 = xnode "FPGA I/O Method Node"("FPGA I/O In"=refnum<k21> "Connector0/DIO2" ("APD 2 DO"), "Timeout"=-1) -> ()  [unwired: 2 out]
          }
          frame #1 {
            n671 = local read "APD3 int gate"() -> (w1272:bool)
            n672 = case shown="True" w1272 {
              frame False {
              }
              frame True {
                n673 = local read "APD3 out state"() -> (w1273:bool)
                n674 = case shown="True" w1273 {
                  frame False {
                    n675 = local read "APD 3 Counts 0"() -> (w1275:u32)
                    n676 = Increment(x=w1275) -> (x+1=→"APD 3 Counts 0":u32)
                  }
                  frame True {
                    n677 = local read "APD 3 Counts 1"() -> (w1277:u32)
                    n678 = Increment(x=w1277) -> (x+1=→"APD 3 Counts 1":u32)
                  }
                }
              }
            }
          }
        }
      }
    }
    frame Enabled {
    }
  }
  n679 = disable-structure shown="Disabled" {
    disable-tunnel: w7 -> [w1279 _]
    disable-tunnel: w4 -> [w1278 _]
    frame Disabled {
      n680 = while "APD 3 Gating" {
        shift-right: [w1283] -> _
        shift-left: w1278 -> [w1288]
        shift-right: [w1282] -> _
        shift-left: w1279 -> [w1280]
        stop <- FALSE stop-if-true
        n681 = flat-sequence {
          tunnel: w1288 -> [w1291]
          tunnel: [w1292] -> w1286
          tunnel: [w1291] -> w1284
          tunnel: [w1290] -> w1281
          tunnel: w1280 -> [w1290]
          tunnel: [w1295] -> w1287
          tunnel: w1286 -> [w1295]
          tunnel: [w1294] -> w1285
          tunnel: w1284 -> [w1294]
          tunnel: w1281 -> [w1293]
          tunnel: [w1316] -> w1283
          tunnel: w1287 -> [w1327]
          tunnel: w1285 -> [w1324]
          tunnel: [w1296] -> w1282
          frame #0 {
            n682 = call "Loop Timer15"("Count(Ticks)"=w1291) -> ("Tick Count(Ticks)"=w1292:u16)
          }
          frame #1 {
            # "Signal maybe then sent through \na transistor before APD"
            n683 = xnode "FPGA I/O Node"("Connector0/DIO12"=w1293, "Connector0/DIO13"=w1293, "Connector0/DIO14"=w1293, "Connector0/DIO15"=w1293) -> ()  [unwired: 4 in, 4 out]
            "APD3 int gate" <- w1293
          }
          frame #2 {
            n684 = local read "APD Gate OFF Count"() -> (w1301:u16)
            n685 = local read "APD Gate ON Count"() -> (w1302:u16)
            n686 = feedback #54(TRUE) -> (w1321:bool)
            n687 = feedback-in #55(w1327) -> ()
            n688 = feedback #55(w1327) -> (w1326:u16)
            n689 = Not(x=w1321) -> (.not. x?=w1319:bool)
            n690 = feedback-in #54(w1319) -> ()
            n691 = Subtract(x=w1327, y=w1326) -> (x-y=w1325:u16)
            n692 = Select(t=w1302, s=w1319, f=w1301) -> (s? t:f=w1323:u16)
            n693 = Subtract(x=w1325, y=w1324) -> (x-y=w1304:u16)
            n694 = Subtract(x=w1323, y=w1304) -> (x-y=w1315:u16)
            n695 = Number To Boolean Array(number=w1304) -> (Boolean array=w1305:bool[])
            n696 = Or Array Elements(Boolean array=w1305) -> (logical OR=w1303:bool)
            n697 = Boolean To (0,1)(Boolean=w1303) -> (0, 1=w1310:i16)
            n698 = Boolean To (0,1)(Boolean="+ phase (APD 3 Gate)") -> (0, 1=w1313:i16)
            n699 = To Unsigned Byte Integer(number=w1310) -> (unsigned 8bit integer=w1307:u8)
            n700 = Multiply(x=w1313, y="Phase count adjustment (APD 3 Gate)") -> (x*y=w1311:i16)
            n701 = feedback #56(u8 0) -> (w1308:u8)
            n702 = Add(x=w1307, y=w1308) -> (x+y=w1306:u8)
            "APD 3 Gate Late Counter" <- w1306
            n703 = feedback-in #56(w1306) -> ()
            n704 = Add(x=w1315, y=w1311) -> (x+y=w1316:u16)
            n705 = feedback #57(i16 0) -> (w1318:i16)
            n706 = Subtract(x=w1318, y=w1311) -> (x-y=w1317:i16)
            "APD 3 Gate Relative Phase" <- w1317
            n707 = feedback-in #57(w1317) -> ()
            n708 = local read "APD Gate Operating Mode"() -> (w1300:u8)
            n709 = case shown="2" w1300 {
              tunnel: [TRUE FALSE w1330] -> w1297
              tunnel: w1321 -> [_ _ w1330]
              frame 0, Default {
              }
              frame 1 {
              }
              frame 2 {
              }
            }
            n710 = local read "Invert APD Gate"() -> (w1299:bool)
            n711 = Not(x=w1297) -> (.not. x?=w1298:bool)
            n712 = Select(t=w1298, s=w1299, f=w1297) -> (s? t:f=w1296:bool)
          }
        }
      }
    }
    frame Enabled {
    }
  }
  n713 = disable-structure shown="Disabled" {
    disable-tunnel: w5 -> [w1332 _]
    disable-tunnel: w4 -> [w1331 _]
    frame Disabled {
      n714 = while "633 nm red  fluorescent laser interlacing (DO to IA 633 nm AOM ME amp)." {
        shift-right: [w1336] -> _
        shift-left: w1331 -> [w1341]
        shift-right: [w1335] -> _
        shift-left: w1332 -> [w1333]
        stop <- FALSE stop-if-true
        n715 = flat-sequence {
          tunnel: w1341 -> [w1344]
          tunnel: [w1345] -> w1339
          tunnel: [w1344] -> w1337
          tunnel: [w1343] -> w1334
          tunnel: w1333 -> [w1343]
          tunnel: [w1348] -> w1340
          tunnel: w1339 -> [w1348]
          tunnel: [w1347] -> w1338
          tunnel: w1337 -> [w1347]
          tunnel: w1334 -> [w1346]
          tunnel: [w1357] -> w1336
          tunnel: w1340 -> [w1377]
          tunnel: w1338 -> [w1374]
          tunnel: [w1366] -> w1335
          frame #0 {
            n716 = call "Loop Timer11"("Count(Ticks)"=w1344) -> ("Tick Count(Ticks)"=w1345:u16)
          }
          frame #1 {
            # "Then to PRL 440 amp"
            n717 = xnode "FPGA I/O Node"("Connector1/DIO32"=w1346) -> ()  [unwired: 1 in, 1 out]
          }
          frame #2 {
            n718 = feedback-in #58(w1377) -> ()
            n719 = feedback #58(w1377) -> (w1376:u16)
            n720 = Subtract(x=w1377, y=w1376) -> (x-y=w1375:u16)
            n721 = Subtract(x=w1375, y=w1374) -> (x-y=w1350:u16)
            n722 = Number To Boolean Array(number=w1350) -> (Boolean array=w1351:bool[])
            n723 = Or Array Elements(Boolean array=w1351) -> (logical OR=w1349:bool)
            n724 = Boolean To (0,1)(Boolean="+ phase (RI)") -> (0, 1=w1362:i16)
            n725 = Multiply(x=w1362, y="Phase count adjustment (RI)") -> (x*y=w1359:i16)
            n726 = Boolean To (0,1)(Boolean=w1349) -> (0, 1=w1356:i16)
            n727 = To Unsigned Byte Integer(number=w1356) -> (unsigned 8bit integer=w1353:u8)
            n728 = feedback #59(i16 0) -> (w1360:i16)
            n729 = feedback #60(u8 0) -> (w1354:u8)
            n730 = Add(x=w1353, y=w1354) -> (x+y=w1352:u8)
            "RI Late Counter" <- w1352
            n731 = feedback-in #60(w1352) -> ()
            n732 = Subtract(x=w1360, y=w1359) -> (x-y=w1358:i16)
            "RI Relative phase" <- w1358
            n733 = feedback-in #59(w1358) -> ()
            n734 = feedback #61(TRUE) -> (w1369:bool)
            n735 = case shown="2" "Red Laser Operating Mode" {
              tunnel: [TRUE FALSE w1383] -> w1366
              tunnel: w1369 -> [_ _ w1380]
              frame 0, Default {
              }
              frame 1 {
              }
              frame 2 {
                n736 = Not(x=w1380) -> (.not. x?=w1382:bool)
                n737 = Select(t=w1382, s="Invert RI", f=w1380) -> (s? t:f=w1383:bool)
              }
            }
            n738 = Not(x=w1369) -> (.not. x?=w1365:bool)
            n739 = Select(t="Red interlace ON count", s=w1365, f="Red interlace OFF count") -> (s? t:f=w1371:u16)
            n740 = Subtract(x=w1371, y=w1350) -> (x-y=w1363:u16)
            n741 = Add(x=w1363, y=w1359) -> (x+y=w1357:u16)
            n742 = feedback-in #61(w1365) -> ()
          }
        }
      }
    }
    frame Enabled {
    }
  }
  n743 = disable-structure shown="Disabled" {
    disable-tunnel: w4 -> [w1384 _]
    frame Disabled {
      n744 = while "Blue fluorescent laser interlacing (AO control direct to laser)." {
        shift-right: [w1391] -> _
        shift-left: w1384 -> [w1394]
        shift-right: [w1388] -> _
        shift-left: i16 0 -> [w1386]
        stop <- FALSE stop-if-true
        n745 = flat-sequence {
          tunnel: w1394 -> [w1397]
          tunnel: [w1398] -> w1393
          tunnel: [w1397] -> w1392
          tunnel: [w1396] -> w1387
          tunnel: w1386 -> [w1396]
          tunnel: [w1401] -> w1390
          tunnel: w1393 -> [w1401]
          tunnel: [w1400] -> w1389
          tunnel: w1392 -> [w1400]
          tunnel: w1387 -> [w1399]
          tunnel: [w1411] -> w1391
          tunnel: [w1427] -> w1388
          tunnel: w1390 -> [w1439]
          tunnel: w1389 -> [w1436]
          frame #0 {
            n746 = call "Loop Timer13"("Count(Ticks)"=w1397) -> ("Tick Count(Ticks)"=w1398:u16)
          }
          frame #1 {
            n747 = xnode "FPGA I/O Node"("Connector0/AO3"=w1399) -> ()  [unwired: 1 in, 1 out]
          }
          frame #2 {
            n748 = Subtract(x="Blue OFF count (AO)", y="Blue current ON count adj (AO)") -> (x-y=w1420:u16)
            n749 = feedback-in #62(w1439) -> ()
            n750 = feedback #62(w1439) -> (w1438:u16)
            n751 = Add(x="Blue current ON count adj (AO)", y="Blue ON count (AO)") -> (x+y=w1421:u16)
            n752 = Subtract(x=w1439, y=w1438) -> (x-y=w1437:u16)
            n753 = Subtract(x=w1437, y=w1436) -> (x-y=w1404:u16)
            n754 = Number To Boolean Array(number=w1404) -> (Boolean array=w1405:bool[])
            n755 = Boolean To (0,1)(Boolean="+ phase (BI AO)") -> (0, 1=w1417:i16)
            n756 = Or Array Elements(Boolean array=w1405) -> (logical OR=w1403:bool)
            n757 = Boolean To (0,1)(Boolean=w1403) -> (0, 1=w1410:i16)
            n758 = Multiply(x=w1417, y="Phase count adjustment (BI AO)") -> (x*y=w1413:i16)
            n759 = To Unsigned Byte Integer(number=w1410) -> (unsigned 8bit integer=w1406:u8)
            n760 = feedback #63(u8 0) -> (w1408:u8)
            n761 = Add(x=w1406, y=w1408) -> (x+y=w1407:u8)
            "BI Late Counter (AO)" <- w1407
            n762 = feedback-in #63(w1407) -> ()
            n763 = feedback #64(i16 0) -> (w1414:i16)
            n764 = Subtract(x=w1414, y=w1413) -> (x-y=w1412:i16)
            "BI Relative phase (AO)" <- w1412
            n765 = feedback-in #64(w1412) -> ()
            n766 = feedback #65(TRUE) -> (w1431:bool)
            n767 = case shown="2" "BI Operating Mode (AO)" {
              tunnel: [TRUE FALSE w1455] -> w1422
              tunnel: w1431 -> [_ _ w1452]
              frame 0, Default {
              }
              frame 1 {
              }
              frame 2 {
                n768 = Not(x=w1452) -> (.not. x?=w1454:bool)
                n769 = Select(t=w1454, s="Invert BI (AO)", f=w1452) -> (s? t:f=w1455:bool)
              }
            }
            n770 = And(x=w1422, y="Blue FB On/Off") -> (x .and. y?=w1423:bool)
            n771 = case shown="True" w1423 {
              tunnel: "BI Current Out" -> [w1440 _]
              tunnel: [w1440 w1442] -> w1426
              frame False {
              }
              frame True {
                n772 = local read "Blue Intensity"() -> (w1441:i16)
                n773 = Bundle("P5"="P5", "I5"="I5", "D5"="D5") -> (w1443:cluster{"P5":i16, "I5":i16, "D5":i16})  [unwired: 1 in]
                n774 = call "Slower PID.vi"("process variable"=w1441, "reset?"="Blue FB Reset", "setpoint"="Blue FB Setpoint", "PID gains (x 2^8)"=w1443, "output range"=cluster{"output high":i16, "output low":i16} {"output high"=32767, "output low"=0} ("Green FB output range")) -> ("output"=w1442:i16)  [unwired: 10 out]
              }
            }
            n775 = Not(x=w1431) -> (.not. x?=w1428:bool)
            n776 = Select(t=w1421, s=w1428, f=w1420) -> (s? t:f=w1433:u16)
            n777 = Subtract(x=w1433, y=w1404) -> (x-y=w1415:u16)
            n778 = Add(x=w1415, y=w1413) -> (x+y=w1411:u16)
            n779 = feedback-in #65(w1428) -> ()
            n780 = Boolean To (0,1)(Boolean=w1422) -> (0, 1=w1402:i16)
            n781 = Multiply(x=w1402, y=w1426) -> (x*y=w1427:i16)
          }
        }
      }
    }
    frame Enabled {
    }
  }
  n782 = disable-structure shown="Disabled" {
    disable-tunnel: w5 -> [w1457 _]
    disable-tunnel: w4 -> [w1456 _]
    frame Disabled {
      n783 = while "473 nm blue  fluorescent laser interlacing (DO to blue laser digital control input)." {
        shift-right: [w1461] -> _
        shift-left: w1456 -> [w1466]
        shift-right: [w1460] -> _
        shift-left: w1457 -> [w1458]
        stop <- FALSE stop-if-true
        n784 = flat-sequence {
          tunnel: w1466 -> [w1469]
          tunnel: [w1470] -> w1464
          tunnel: [w1469] -> w1462
          tunnel: [w1468] -> w1459
          tunnel: w1458 -> [w1468]
          tunnel: [w1473] -> w1465
          tunnel: w1464 -> [w1473]
          tunnel: [w1472] -> w1463
          tunnel: w1462 -> [w1472]
          tunnel: w1459 -> [w1471]
          tunnel: [w1482] -> w1461
          tunnel: w1465 -> [w1502]
          tunnel: w1463 -> [w1499]
          tunnel: [w1491] -> w1460
          frame #0 {
            n785 = call "Loop Timer14"("Count(Ticks)"=w1469) -> ("Tick Count(Ticks)"=w1470:u16)
          }
          frame #1 {
            n786 = xnode "FPGA I/O Node"("Connector1/DIO28"=w1471) -> ()  [unwired: 1 in, 1 out]
          }
          frame #2 {
            n787 = feedback-in #66(w1502) -> ()
            n788 = feedback #66(w1502) -> (w1501:u16)
            n789 = Subtract(x=w1502, y=w1501) -> (x-y=w1500:u16)
            n790 = Subtract(x=w1500, y=w1499) -> (x-y=w1475:u16)
            n791 = Number To Boolean Array(number=w1475) -> (Boolean array=w1476:bool[])
            n792 = Or Array Elements(Boolean array=w1476) -> (logical OR=w1474:bool)
            n793 = Boolean To (0,1)(Boolean="+ phase (BI D)") -> (0, 1=w1487:i16)
            n794 = Multiply(x=w1487, y="Phase count adjustment (BI D)") -> (x*y=w1484:i16)
            n795 = Boolean To (0,1)(Boolean=w1474) -> (0, 1=w1481:i16)
            n796 = To Unsigned Byte Integer(number=w1481) -> (unsigned 8bit integer=w1478:u8)
            n797 = feedback #67(i16 0) -> (w1485:i16)
            n798 = feedback #68(u8 0) -> (w1479:u8)
            n799 = Add(x=w1478, y=w1479) -> (x+y=w1477:u8)
            "Blue Late Counter (D)" <- w1477
            n800 = feedback-in #68(w1477) -> ()
            n801 = Subtract(x=w1485, y=w1484) -> (x-y=w1483:i16)
            "BI Relative phase (D)" <- w1483
            n802 = feedback-in #67(w1483) -> ()
            n803 = feedback #69(TRUE) -> (w1494:bool)
            n804 = case shown="2" "Blue Laser Operating Mode (D)" {
              tunnel: [TRUE FALSE w1508] -> w1491
              tunnel: w1494 -> [_ _ w1505]
              frame 0, Default {
              }
              frame 1 {
              }
              frame 2 {
                n805 = Not(x=w1505) -> (.not. x?=w1507:bool)
                n806 = Select(t=w1507, s="Invert BI (D)", f=w1505) -> (s? t:f=w1508:bool)
              }
            }
            n807 = Not(x=w1494) -> (.not. x?=w1490:bool)
            n808 = Select(t="Blue interlace ON count (D)", s=w1490, f="Blue interlace OFF count (D)") -> (s? t:f=w1496:u16)
            n809 = Subtract(x=w1496, y=w1475) -> (x-y=w1488:u16)
            n810 = Add(x=w1488, y=w1484) -> (x+y=w1482:u16)
            n811 = feedback-in #69(w1490) -> ()
          }
        }
      }
    }
    frame Enabled {
    }
  }
